vi "V1.1_UI.vi"() -> ()   [LabVIEW 2018]
uses:
  <vilib>/MakerHub/LINX/Private/Type Defs/LINX Ref.ctl
  <vilib>/MakerHub/LINX/Private/Type Defs/Platform.ctl
  <vilib>/MakerHub/LINX/Private/Type Defs/Interface.ctl
  <vilib>/MakerHub/LINX/Private/Device/Type Defs/LINX Device Config.ctl
  <vilib>/MakerHub/LINX/Private/Device/Type Defs/TCP Config.ctl
  <vilib>/MakerHub/LINX/Private/Device/Type Defs/Channels.ctl
  <vilib>/MakerHub/LINX/Public/Peripherals/Digital/Digital Write N Chans.vi
  <vilib>/MakerHub/LINX/Private/Local IO/LinxDigitalWrite.vi
  <vilib>/MakerHub/LINX/Public/Utilities/Check Channel.vi
  <vilib>/MakerHub/LINX/Public/Utilities/Open Serial.vi
  <vilib>/MakerHub/LINX/Private/Utilties/Generate Error.vi
  lib/Olympus IX BX Series/Olympus IX BX Series.lvlib
  <vilib>/MakerHub/LINX/LMH-LINX.lvlib
  lib/SOLA/LabVIEW 2015 Library (32bit)/LumencorDLL32/LumencorDLL32.lvlib
  lib/ANDOR/Andor SDK/AndorSDK.lvlib
  <vilib>/vision/NI_Vision_Development_Module.lvlib
  <userlib>/Tango_DLL/Tango_DLL.lvlib
  <userlib>/Andor SDK/Andor SDK.lvlib
  <vilib>/MakerHub/LINX/Private/Device/Device.lvlib
panel:
  in  "Export List":bool
  in  "Colormap":u16(ring) items=["Grey", "Hot"]
  in  "Format":u16(ring)=6
  in  "Path":path
  in  "Save Image":bool
  out "error out":errorcluster
  out "SOLA ID":u32
  out "TANGO ID":i32
  out "LINX Resource":T1={"IO"=enum."Remote", "Interface"=enum."TCP", "LINX Device Config"={"Interface"=enum."Serial", "COM Port"="COM13", "TCP Configuration"={"IP Address"="", "Port"=0}, "Device Family"=1, "Device ID"=1, "Device Name"="myRIO-1900", "TCP Ref"=refnum, "Channels"={"DI"=[0, 1, 2, 3, 4, 5, 6, 7, 8, 9, 10, 11, 12, 13, 14, 15, 16, 17, 18, 19, 20, 21, 22, 23, 24, 25, 26, 27, 28, 29, 30, 31, 32, 33, 34, 35, 36, 37, 38, 39, 40, 41, 42, 43, 44, 45, 46], "DO"=[0, 1, 2, 3, 4, 5, 6, 7, 8, 9, 10, 11, 12, 13, 14, 15, 16, 17, 18, 19, 20, 21, 22, 23, 24, 25, 26, 27, 28, 29, 30, 31, 32, 33, 34, 35, 36, 37, 38, 39, 40, 41, 42, 43, 44, 45, 46], "AI"=[0, 1, 2, 3, 4, 5, 6, 7, 8, 9, 10, 11], "AO"=[], "PWM"=[3, 5, 6, 9, 10], "QE"=[], "UART"=[0, 1], "I2C 2"=[0], "SPI"=[0], "CAN"=[], "Servo"=[], "AI Ref (V)"=0.0, "AI Resolution (Bits)"=0, "AO Ref (V)"=0.0, "AO Resolution (Bits)"=0}}}
  out "elements":cluster{"Button":string, "Value":dbl}[](array[cluster])
  in  "Filter":u16(ring) items=["UV ", "CFP", "GFP", "YFP", "RFP", "BF (empty)"]
  in  "Exposure":sgl=50.0 format="%#_g ms"
  out "exposure out":sgl
  out "accumulate out":sgl
  out "kinetic out":sgl
  out "Camera Temperature":sgl format="%.2f °C"
  in  "Single/\nMultiring?":bool
  in  "Image Name":string="TestIMG"
  out "Acq. Error Array":cluster{i32, string}[](array[cluster])
  in  "Live Mode":bool
  in  "Single Image":bool
  in  "Calibrate at Startup":bool
  out "keys pressed":T7(array[ring])
  in  "Position List":i32[](listbox)
  in  "Down":bool
  in  "Left":bool
  in  "Up":bool
  in  "Right":bool
  in  "Clear Last Pos":bool
  in  "Save Pos":bool
  out "Tango Success":bool
  in  "TANGO COM Port":refnum<visa-resource-name>="COM4"
  in  "SOLA COM Port":refnum<visa-resource-name>="COM5"
  in  "Valve Port (Arduino)":refnum<visa-resource-name>="COM7"
  in  "IX 81 Port":refnum<visa-resource-name>="IX2-UCB"
  out "Tango Connection\n Error":i32
  out "Y Limits":dbl[](array[numeric]) caption="Y Limits [µm]" format="%#_12f"
  out "X Limits":dbl[](array[numeric]) caption="X Limits [µm]" format="%#_10f"
  in  "TangoStep":dbl=100.0 caption="Step Width [µm]" min=0.0 format="%#_6f"
  out "Position":dbl[](array[numeric]) caption="Position [µm]" format="%#_12f"
  in  "Focus [um]":dbl format="%.3f"
  out "Upper Limit":dbl
  out "Lower Limit":dbl
  in  "Light Source":u16(ring) items=["BF - Lamp", "SOLA"]
  in  "Intensity [%]":dbl(slide) scale=0.0..100.0 scale format="%.1f"
  in  "Prism Position (1: Bi)":enum16{"Bi", "Side"}(ring)=enum."Side"
  in  "Objective":enum16{"x 4", "x 10", "x 20", "x 40", "x 100"}(ring)=enum."x 10"
  in  "Shutter":bool
  in  "Enable Lamp":bool
  in  "Lamp Type (0: Transmitted)":enum16{"Transmitted", "Reflected"}(ring)
  out "Info":string caption="String"
  out "Image":T8(plugin-control)
  in  "Flush\nReagent":u16
  in  "Flush":bool
  in  "Pump Cycles":dbl=20.0
  in  "Frequency":dbl=50.0 format="%#_3f"
  in  "Pump On":bool
  in  "Feed On":bool
  in  "Feed Cycles":i32=20
  in  "Feed\nReagent":u16=2
  in  "Ring":u16
  in  "All Rings":bool
  in  "stop":bool
  # "Initialization"
  # "Stage"
  # "X"
  # "Y"
  # "min"
  # "min"
  # "max"
  # "max"
  # "S"
  # "M"
  # "Microscope"
  # "Valve Functions"
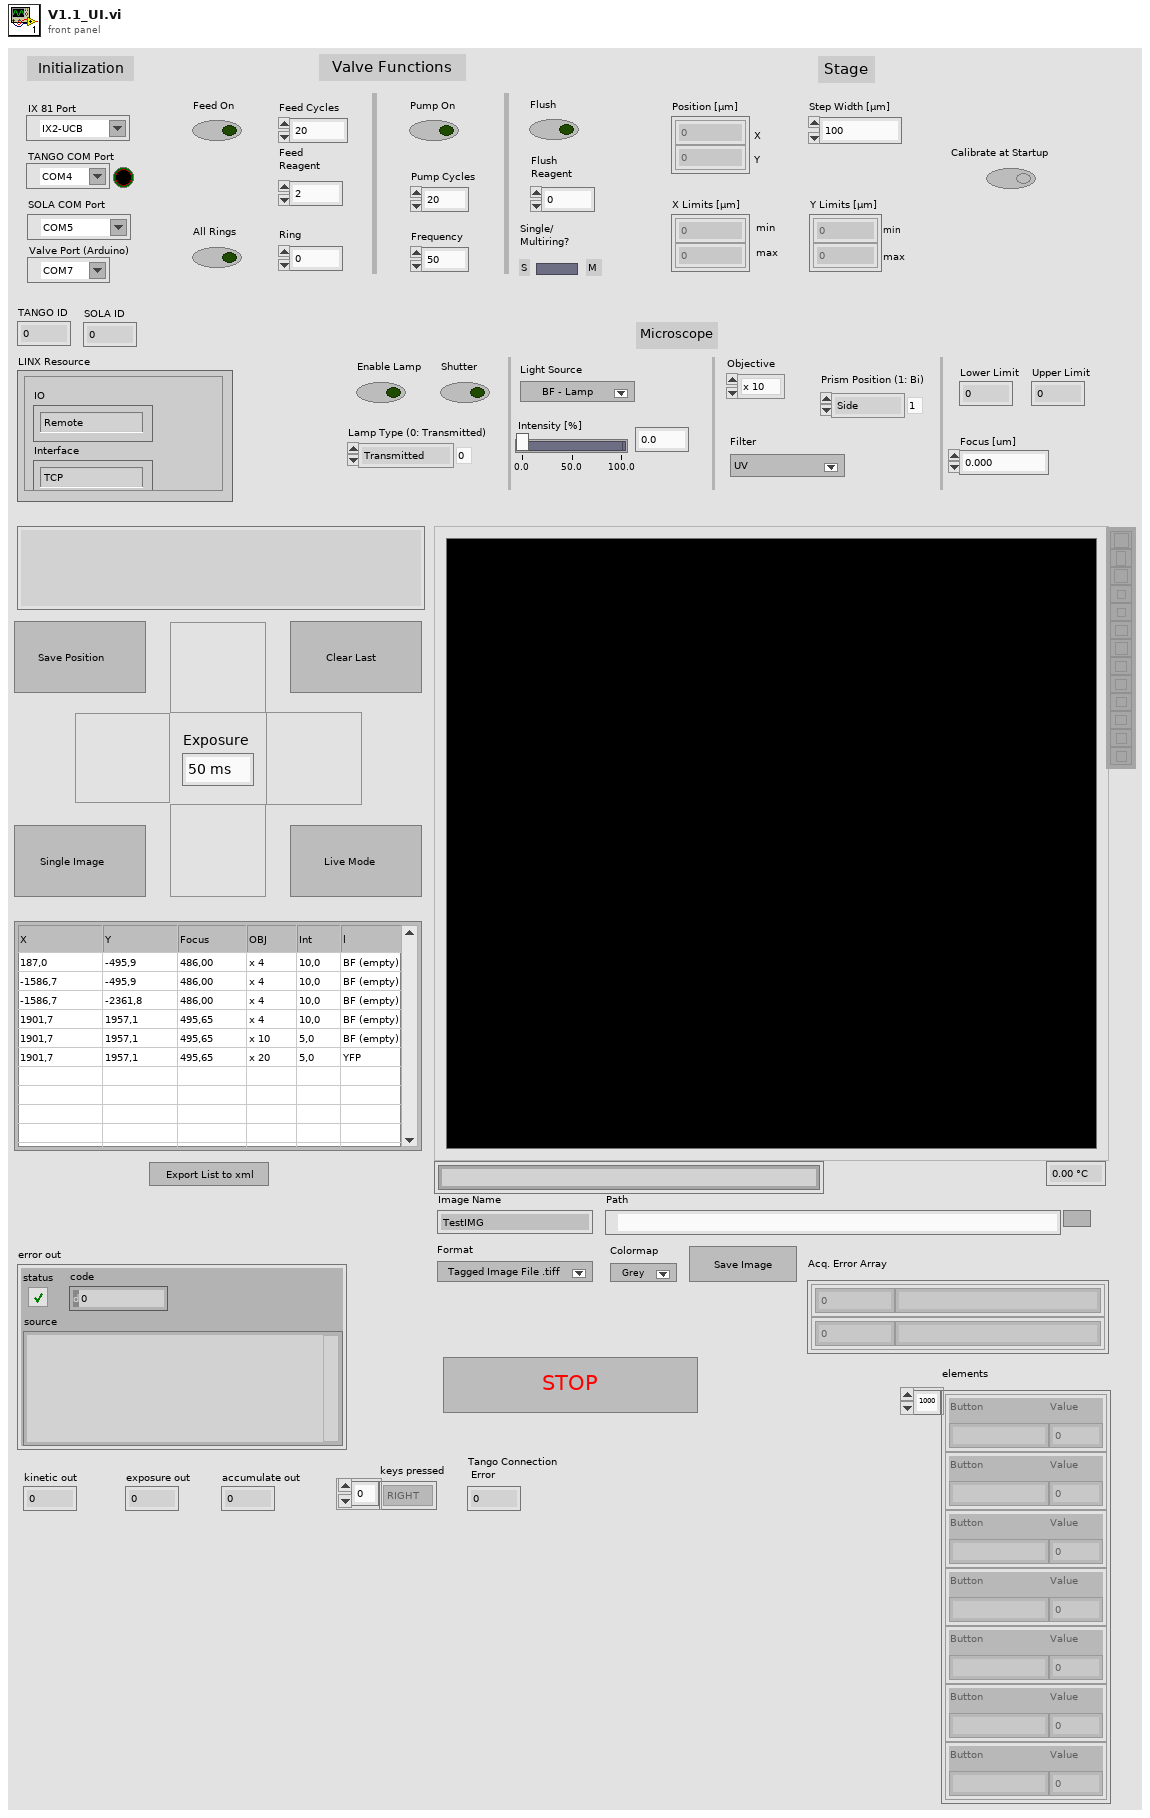
[diagram p1: front panel]
types:
  T1 = typedef "LMH-LINX.lvlib/LINX Ref.ctl" = cluster{"IO":T2, "Interface":T3, "LINX Device Config":T4}
  T2 = typedef "LMH-LINX.lvlib/Platform.ctl" = enum16{"Remote", "Local"}
  T3 = typedef "LMH-LINX.lvlib/Interface.ctl" = enum16{"Serial", "TCP"}
  T4 = typedef "LMH-LINX.lvlib/Device.lvlib/LINX Device Config.ctl" = cluster{"Interface":T3, "COM Port":refnum<visa-resource-name>, "TCP Configuration":T5, "Device Family":u8, "Device ID":u8, "Device Name":string, "TCP Ref":refnum<k5>, "Channels":T6}
  T5 = typedef "LMH-LINX.lvlib/Device.lvlib/TCP Config.ctl" = cluster{"IP Address":string, "Port":u16}
  T6 = typedef "LMH-LINX.lvlib/Channels.ctl" = cluster{"DI":u8[], "DO":u8[], "AI":u8[], "AO":u8[], "PWM":u8[], "QE":u8[], "UART":u8[], "I2C 2":u8[], "SPI":u8[], "CAN":u8[], "Servo":u8[], "AI Ref (V)":dbl, "AI Resolution (Bits)":u8, "AO Ref (V)":dbl, "AO Resolution (Bits)":u8}
  T7 = enum16{"0", "1", "2", "3", "4", "5", "6", "7", "8", "9", "A", "B", "C", "D", "E", "F", "G", "H", "I", "J", "K", "L", "M", "N", "O", "P", "Q", "R", "S", "T", "U", "V", "W", "X", "Y", "Z", "F1", "F2", "F3", "F4", "F5", "F6", "F7", "F8", "F9", "F10", "F11", "F12", "F13", "F14", "F15", "ADD", "BACK", "BACKSLASH", "CAPITAL", "COMMA", "DECIMAL", "DELETE", "DIVIDE", "DOWN", "END", "EQUALS", "ESCAPE", "GRAVE (`)", "HOME", "INSERT", "LBRACKET", "LCONTROL", "LEFT", "L ALT", "LSHIFT", "LWIN", "MINUS", "MULTIPLY", "NEXT", "NUMLOCK", "NUMPAD_0", "NUMPAD_1", "NUMPAD_2", "NUMPAD_3", "NUMPAD_4", "NUMPAD_5", "NUMPAD_6", "NUMPAD_7", "NUMPAD_8", "NUMPAD_9", "PAUSE", "PERIOD", "PRIOR (PG UP)", "RBRACKET", "RCONTROL", "RETURN", "RIGHT", "R ALT", "RSHIFT", "RWIN", "SCROLL", "SEMICOLON", "SLASH", "SPACE", "SUBTRACT", "TAB", "UP", "ENTER (num pad)", "' (quote)"}[]
  T8 = typedef "IMAQ Image.ctl" = refnum<image>
  T9 = enum8{"Enabled", "Disabled", "Disabled and Grayed Out"}
  T10 = enum32{"UV", "CFP", "GFP", "YFP", "RFP", "BF (empty)"}
  T11 = typedef "Image Type" = u32
  T12 = cluster{"pdX out":dbl, "pdY out":dbl, dbl, string, string, "Intensity [%]":dbl}
  T13 = cluster{"pdX out":dbl, "pdY out":dbl, dbl, string, string, "Intensity [%]":dbl}[]
  T14 = cluster{string, "NewVal":enum16{"x 4", "x 10", "x 20", "x 40", "x 100"}}
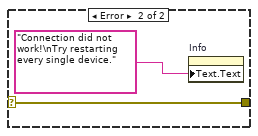
[diagram p2: hidden frame]
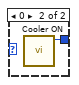
[diagram p3: hidden frame]
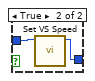
[diagram p4: hidden frame]
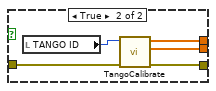
[diagram p5: hidden frame]
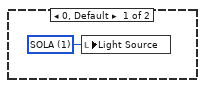
[diagram p6: hidden frame]
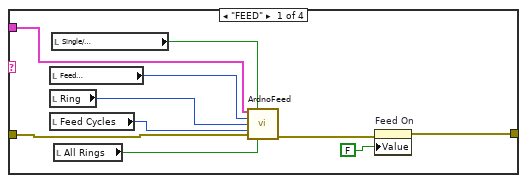
[diagram p7: hidden frame]
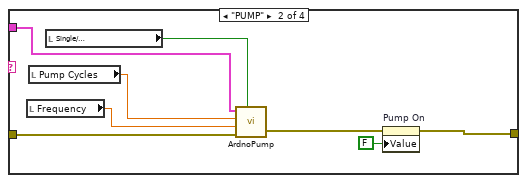
[diagram p8: hidden frame]
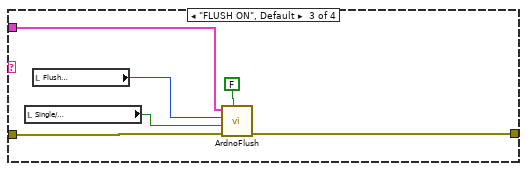
[diagram p9: hidden frame]
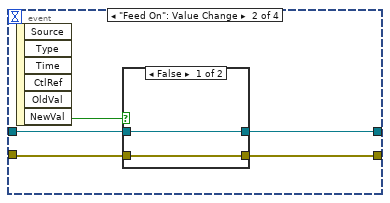
[diagram p10: hidden frame]
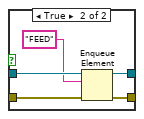
[diagram p11: hidden frame]
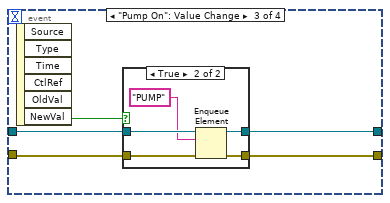
[diagram p12: hidden frame]
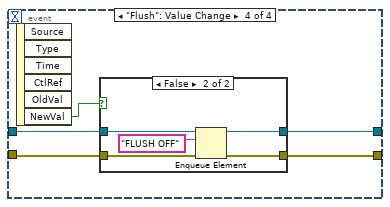
[diagram p14: hidden frame]
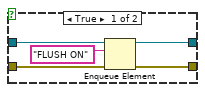
[diagram p15: hidden frame]
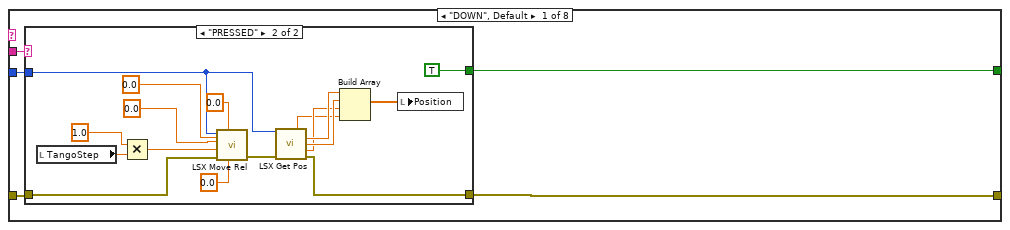
[diagram p16: hidden frame]
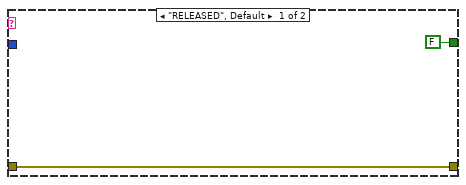
[diagram p17: hidden frame]
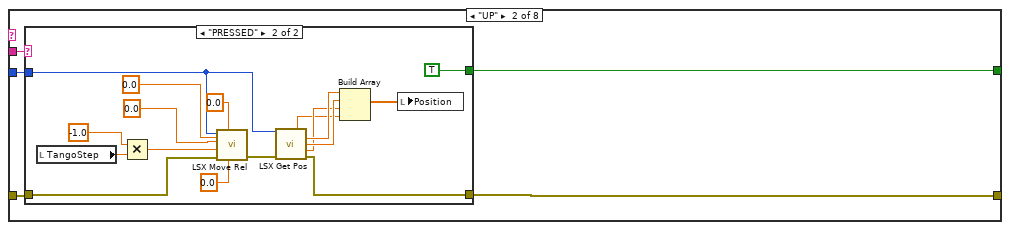
[diagram p18: hidden frame]
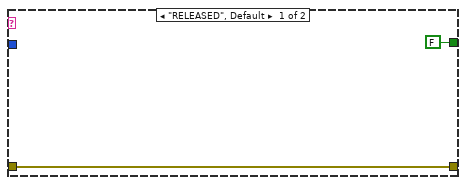
[diagram p19: hidden frame]
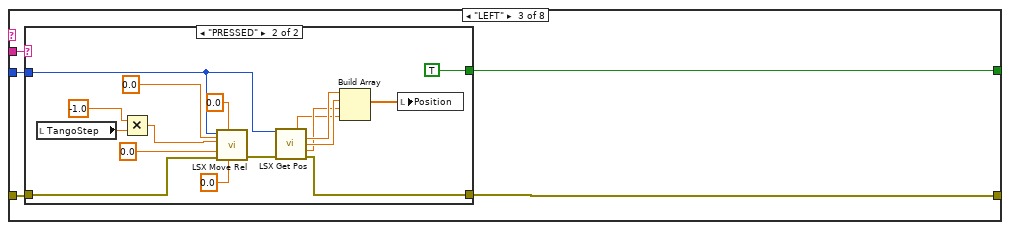
[diagram p20: hidden frame]
diagram:
  n1 = flat-sequence {
    tunnel: [w15] -> w2
    tunnel: w2 -> [w119]
    tunnel: [w115] -> w1
    tunnel: w1 -> [w228]
    tunnel: [w233] -> w5
    tunnel: w5 -> [w1109]
    tunnel: [w1108] -> w4
    tunnel: w4 -> [w1135]
    tunnel: [w1135] -> w3
    frame #0 {
      # "Connection String"
      n2 = local write "Info"("Connecting..." ("Info")) -> ()
    }
    frame #1 {
      w29 = 2  # Device Number (1: Condensor, Objective Lamp,Shutter 2: Z-Motion, Autofocus)
      w32 = 1  # Device Number (1: Condensor, Objective Lamp,Shutter 2: Z-Motion, Autofocus)
      # "Establishing Connections To All Devices"
      n3 = local read "Valve Port (Arduino)"() -> (w27:refnum<visa-resource-name>)
      n4 = property on="SOLA COM Port" class="VISAName"() -> ("Text.Text"=w24:string)  [unwired: 2 in, 2 out]
      n5 = local read "TANGO COM Port"() -> (w11:refnum<visa-resource-name>)
      n6 = local read "IX 81 Port"() -> (w28:refnum<visa-resource-name>)
      n7 = Scan From String(format string="COM%d", input string=w24) -> (output 1=w22:i32)  [unwired: 3 in, 3 out]
      n8 = Decrement(x=w22) -> (x-1=w21:i32)
      n9 = call-poly <vilib>:"Open.vi"("Serial Port"=w27) -> ("Error Out"=w25:errorcluster, "LINX Resource"=→"LINX Resource":T1)  [unwired: 8 in, 1 out]
      n10 = call "Initialize.vi"("VISA Resource Name"=w28) -> ("VISA Resource Name Out"=w33:refnum<visa-resource-name>, "error out"=w34:errorcluster)  [unwired: 13 in]
      n11 = call "lm Init.vi"("LETypeStr"="SOLA", "ComPort"=w21) -> ("error out"=w19:errorcluster, "function return"=→"SOLA ID":u32)  [unwired: 7 in, 1 out]
      n12 = call "AndorCreaterErrorCluster.vi"() -> ("Array"=w7:cluster{i32, string}[])  [unwired: 11 in]
      n13 = call "TangoConnect.vi"("Tango Com"=w11) -> ("error out"=w10:errorcluster, "success"=w8:bool, "plLSID out"=→"TANGO ID":i32)  [unwired: 7 in, 1 out]
      n14 = call "Initialize.vi"("dir"="C:\\Users\\e14user\\Documents\\LabVIEW software\\GitRepo\\lib\\ANDOR\\Libraries") -> ("function return"=w17:u32)  [unwired: 9 in, 1 out]
      n15 = call "Login Device.vi"("error in (no error)"=w34, "Device Number (1)"=w32, "VISA Resource Name"=w33) -> ("error out"=w30:errorcluster, "VISA Resource Name Out"=w31:refnum<visa-resource-name>)  [unwired: 7 in]
      n16 = call "Login Device.vi"("error in (no error)"=w30, "Device Number (1)"=w29, "VISA Resource Name"=w31) -> ("error out"=w26:errorcluster)  [unwired: 7 in, 1 out]
      n17 = local write "Tango Success"(w8) -> ()
      n18 = property on="Tango Success" class="Bool (strict)"("Colors [4]"=cluster{u32, u32}[] [{16711680, 0}, {65280, 0}, {6710886, 0}, {6710886, 0}]) -> ()  [unwired: 2 in, 2 out]
      n19 = call "AndorReturn2Error.vi"("Error List"=w7, "Camera return"=w17) -> ("error out"=w16:errorcluster)  [unwired: 8 in, 1 out]
      n20 = Merge Errors(w26, w25, w19, w10, w16) -> (w14:errorcluster)
      n21 = case shown="No Error" w14 {
        selector: w14 -> [w36 w39]
        tunnel: [w36 w39] -> w15
        frame No Error {
          n22 = property on="Info" class="Str"("Text.Text"="Connection finished!") -> ()  [unwired: 2 in, 2 out]
        }
        frame Error {
          n23 = property on="Info" class="Str"("Text.Text"="Connection did not work!\nTry restarting every single device.") -> ()  [unwired: 2 in, 2 out]
        }
      }
    }
    frame #2 {
      w104 = 0  # openingtime
      w102 = 0  # Auto Mode
      w101 = 1  # TTL High to open
      w103 = 0  # closingtime
      w100 = 0  # Internal Trigger
      w98 = 1  # Single Scan
      w99 = 4  # Image Read
      # "Initializing Devices With (Config File)"
      n24 = local read "Calibrate at Startup"() -> (w124:bool)
      n25 = local read "IX 81 Port"() -> (w194:refnum<visa-resource-name>)
      n26 = call "AndorCreaterErrorCluster.vi"() -> ("Array"=w72:cluster{i32, string}[])  [unwired: 11 in]
      n27 = call "Is Cooler On.vi"() -> ("function return"=w87:u32, "iCoolerStatus out"=w88:i32)  [unwired: 10 in]
      n28 = call "lm Color Level.vi"("error in (no error)"=w119, "str_Level"="0", "str_Color"="WHITE") -> ("error out"=w198:errorcluster, "str_Color out"=w199:string)  [unwired: 6 in, 1 out]
      n29 = call "Set Active Objective.vi"("error in (no error)"=w119, "Objective Number (1)"=1, "Device Number (1)"=1, "VISA Resource Name"=w194) -> ("error out"=w141:errorcluster, "VISA Resource Name Out"=w142:refnum<visa-resource-name>)  [unwired: 6 in]
      n30 = call "AndorReturn2Error.vi"("Error List"=w72, "Camera return"=w87) -> ("error out"=w70:errorcluster, "Error List out"=w71:cluster{i32, string}[])  [unwired: 8 in]
      n31 = call "lm Color Enable.vi"("error in (no error)"=w198, "str_State"="OFF", "str_Color"=w199) -> ("error out"=w112:errorcluster)  [unwired: 6 in, 2 out]
      n32 = case shown="False" w124 {
        tunnel: [w207 w214] -> w111
        tunnel: w119 -> [w207 w210]
        tunnel: [dbl[] [0.0, 80674.8] ("Y Limits") w213] -> w122
        tunnel: [dbl[] [0.0, 120822.0] ("X Limits") w212] -> w123
        frame False {
        }
        frame True {
          n33 = local read "TANGO ID"() -> (w211:i32)
          n34 = call "TangoCalibrate.vi"("error in (no error)"=w210, "plLSID in"=w211) -> ("error out"=w214:errorcluster, "X Limits"=w212:dbl[], "Y Limits"=w213:dbl[])  [unwired: 7 in]
        }
      }
      n35 = case shown="1, Default" w88 {
        tunnel: [u32 20002 ("function return") w203] -> w86
        frame 1, Default {
        }
        frame 0 {
          n36 = call "Cooler ON.vi"() -> ("function return"=w203:u32)  [unwired: 11 in]
        }
      }
      n37 = call "OlympusQuery.vi"("error in (no error)"=w141, "String"="SW OFF", "VISA Resource Name In"=w142) -> ("error out"=w145:errorcluster, "VISA Resource Name Out"=w146:refnum<visa-resource-name>)  [unwired: 6 in, 1 out]
      n38 = call "OlympusQuery.vi"("error in (no error)"=w145, "String"="LMPSW?", "VISA Resource Name In"=w146) -> ("error out"=w140:errorcluster, "Result"=w173:string, "VISA Resource Name Out"=w191:refnum<visa-resource-name>)  [unwired: 6 in]
      n39 = call "AndorReturn2Error.vi"("error in (no error)"=w70, "Error List"=w71, "Camera return"=w86) -> ("error out"=w69:errorcluster, "Error List out"=w43:cluster{i32, string}[])  [unwired: 7 in]
      n40 = Equal?(x=w173, y="ON") -> (x = y?=w139:bool)
      n41 = local write "Enable Lamp"(w139) -> ()
      n42 = call "OlympusQuery.vi"("error in (no error)"=w140, "String"="LMP?", "VISA Resource Name In"=w191) -> ("error out"=w137:errorcluster, "Result"=w148:string, "VISA Resource Name Out"=w190:refnum<visa-resource-name>)  [unwired: 6 in]
      n43 = call "Set Temperature.vi"("temperature"=-60) -> ()  [unwired: 10 in, 1 out]
      n44 = Decimal String To Number(string=w148, default (0L)=0.0 ("default (0 I32)")) -> (number=w150:dbl)  [unwired: 1 in, 1 out]
      n45 = local read "LINX Resource"() -> (w121:T1)
      n46 = local write "Y Limits"(w122) -> ()
      n47 = local write "X Limits"(w123) -> ()
      n48 = Divide(x=w150, y=1.2 ("x")) -> (x/y=w138:dbl)
      n49 = local write "Intensity [%]"(w138) -> ()
      n50 = call "ArdnoValve2Linx.vi"("error in (no error)"=w119, "Valve (A1-C8),\n comma separated"="A1,A2,A3,A4,A5,A6,A7,A8,B1,B2,B3,B4,B5,B6,B7,B8,C1,C2,C3,C4,C5,C6,C7,C8" ("Valve (A1-C8),\n comma separated")) -> ("error out"=w118:errorcluster, "Array"=w117:bool[], "Array 2"=w116:i32[])  [unwired: 7 in]
      n51 = call "Get Fastest Recommended VS Speed.vi"() -> ("function return"=w73:u32, "speed out"=w106:sgl, "index out"=w109:i32)  [unwired: 9 in]
      n52 = call "OlympusQuery.vi"("error in (no error)"=w137, "String"="SHUT1?", "VISA Resource Name In"=w190) -> ("error out"=w135:errorcluster, "Result"=w171:string, "VISA Resource Name Out"=w188:refnum<visa-resource-name>)  [unwired: 6 in]
      n53 = call-poly <vilib>:"Digital Write.vi"("Error In"=w118, "Values"=w117, "DO Channels"=w116, "LINX Resource"=w121) -> ("Error Out"=w113:errorcluster)  [unwired: 6 in, 1 out]
      n54 = Equal?(x=w171, y="OUT") -> (x = y?=w136:bool)
      n55 = local write "Shutter"(w136) -> ()
      n56 = call "AndorReturn2Error.vi"("error in (no error)"=w69, "Error List"=w43, "Camera return"=w73) -> ("error out"=w68:errorcluster, "Error List out"=w44:cluster{i32, string}[])  [unwired: 7 in]
      n57 = call "Get VS Speed.vi"() -> ("speed out"=w107:sgl, "function return"=w74:u32)  [unwired: 10 in]
      n58 = call "OlympusQuery.vi"("error in (no error)"=w135, "String"="LMPSEL?", "VISA Resource Name In"=w188) -> ("error out"=w132:errorcluster, "Result"=w169:string, "VISA Resource Name Out"=w133:refnum<visa-resource-name>)  [unwired: 6 in]
      n59 = Greater Or Equal?(x=w106, y=w107) -> (x >= y?=w108:bool)
      n60 = call "AndorReturn2Error.vi"("error in (no error)"=w68, "Error List"=w44, "Camera return"=w74) -> ("error out"=w67:errorcluster, "Error List out"=w45:cluster{i32, string}[])  [unwired: 7 in]
      n61 = Equal?(x=w169, y="DIA") -> (x = y?=w167:bool)
      n62 = Not(x=w167) -> (.not. x?=w166:bool)
      n63 = case shown="False" w108 {
        tunnel: w109 -> [_ w206]
        tunnel: [u32 20002 ("function return") w205] -> w75
        frame False {
        }
        frame True {
          n64 = call "Set VS Speed.vi"("index"=w206) -> ("function return"=w205:u32)  [unwired: 10 in]
        }
      }
      n65 = Boolean To (0,1)(Boolean=w166) -> (0, 1=w134:i16)
      n66 = local write "Lamp Type (0: Transmitted)"(w134) -> ()
      n67 = call "OlympusQuery.vi"("error in (no error)"=w132, "String"="MU?", "VISA Resource Name In"=w133) -> ("error out"=w131:errorcluster, "Result"=w165:string, "VISA Resource Name Out"=w144:refnum<visa-resource-name>)  [unwired: 6 in]
      n68 = call "AndorReturn2Error.vi"("error in (no error)"=w67, "Error List"=w45, "Camera return"=w75) -> ("error out"=w66:errorcluster, "Error List out"=w46:cluster{i32, string}[])  [unwired: 7 in]
      n69 = Decimal String To Number(string=w165) -> (number=w164:i32)  [unwired: 2 in, 1 out]
      n70 = call "Get Temperature F.vi"() -> ("function return"=w76:u32, "temperature out"=w105:sgl)  [unwired: 10 in]
      n71 = Decrement(x=w164) -> (x-1=w143:i32)
      n72 = case shown="5" w143 {
        frame 0, Default {
          w215 = u16 1 items=["BF - Lamp", "SOLA"] ("Light Source")
          n73 = local write "Light Source"(w215) -> ()
        }
        frame 5 {
          w216 = u16 0 items=["BF - Lamp", "SOLA"] ("Light Source")
          n74 = local write "Light Source"(w216) -> ()
        }
      }
      n75 = local write "Filter"(w143) -> ()
      n76 = call "AndorReturn2Error.vi"("error in (no error)"=w66, "Error List"=w46, "Camera return"=w76) -> ("error out"=w65:errorcluster, "Error List out"=w47:cluster{i32, string}[])  [unwired: 7 in]
      n77 = local write "Camera Temperature"(w105) -> ()
      n78 = call "OlympusQuery.vi"("error in (no error)"=w131, "String"="OB?", "VISA Resource Name In"=w144) -> ("error out"=w129:errorcluster, "Result"=w163:string, "VISA Resource Name Out"=w183:refnum<visa-resource-name>)  [unwired: 6 in]
      n79 = Decimal String To Number(string=w163) -> (number=w162:i32)  [unwired: 2 in, 1 out]
      n80 = Decrement(x=w162) -> (x-1=w130:i32)
      n81 = call "Set Read Mode.vi"("mode"=w99) -> ("function return"=w77:u32)  [unwired: 10 in]
      n82 = local write "Objective"(w130) -> ()
      n83 = call "AndorReturn2Error.vi"("error in (no error)"=w65, "Error List"=w47, "Camera return"=w77) -> ("error out"=w64:errorcluster, "Error List out"=w48:cluster{i32, string}[])  [unwired: 7 in]
      n84 = local write "Lower Limit"(10.0 ("Upper Limit")) -> ()
      n85 = call "OlympusQuery.vi"("error in (no error)"=w129, "String"="PRISM?", "VISA Resource Name In"=w183) -> ("error out"=w128:errorcluster, "Result"=w161:string, "VISA Resource Name Out"=w182:refnum<visa-resource-name>)  [unwired: 6 in]
      n86 = Decimal String To Number(string=w161) -> (number=w160:i32)  [unwired: 2 in, 1 out]
      n87 = call "Set Shutter.vi"("openingtime"=w104, "closingtime"=w103, "mode"=w102, "typ"=w101) -> ("function return"=w78:u32)  [unwired: 7 in]
      n88 = Decrement(x=w160) -> (x-1=w127:i32)
      n89 = local write "Prism Position (1: Bi)"(w127) -> ()
      n90 = call "OlympusQuery.vi"("error in (no error)"=w128, "Device Number\n(1: -Condensor\n     - Objective\n     - Lamp\n     - Shutter\n2: - Z-Motion\n   - Autofocus)"=2 ("Device Number\n(1: -Condensor\n     - Objective\n     - Lamp\n     - Shutter\n2: - Z-Motion\n   - Autofocus)"), "String"="FARLMT 10", "VISA Resource Name In"=w182) -> ("error out"=w179:errorcluster, "VISA Resource Name Out"=w180:refnum<visa-resource-name>)  [unwired: 5 in, 1 out]
      n91 = call "AndorReturn2Error.vi"("error in (no error)"=w64, "Error List"=w48, "Camera return"=w78) -> ("error out"=w63:errorcluster, "Error List out"=w49:cluster{i32, string}[])  [unwired: 7 in]
      n92 = local write "Upper Limit"(3000000.0 ("default (0 I32)")) -> ()
      n93 = call "Set Trigger Mode.vi"("mode"=w100) -> ("function return"=w79:u32)  [unwired: 10 in]
      n94 = call "AndorReturn2Error.vi"("error in (no error)"=w63, "Error List"=w49, "Camera return"=w79) -> ("error out"=w62:errorcluster, "Error List out"=w50:cluster{i32, string}[])  [unwired: 7 in]
      n95 = call "OlympusQuery.vi"("error in (no error)"=w179, "Device Number\n(1: -Condensor\n     - Objective\n     - Lamp\n     - Shutter\n2: - Z-Motion\n   - Autofocus)"=2 ("Device Number\n(1: -Condensor\n     - Objective\n     - Lamp\n     - Shutter\n2: - Z-Motion\n   - Autofocus)"), "String"="NEARLMT 3000000", "VISA Resource Name In"=w180) -> ("error out"=w176:errorcluster, "VISA Resource Name Out"=w177:refnum<visa-resource-name>)  [unwired: 5 in, 1 out]
      n96 = call "Set Acquisition Mode.vi"("mode"=w98) -> ("function return"=w80:u32)  [unwired: 10 in]
      n97 = call "OlympusQuery.vi"("error in (no error)"=w176, "Device Number\n(1: -Condensor\n     - Objective\n     - Lamp\n     - Shutter\n2: - Z-Motion\n   - Autofocus)"=2 ("Device Number\n(1: -Condensor\n     - Objective\n     - Lamp\n     - Shutter\n2: - Z-Motion\n   - Autofocus)"), "String"="POS?", "VISA Resource Name In"=w177) -> ("error out"=w154:errorcluster, "Result"=w155:string, "VISA Resource Name Out"=w153:refnum<visa-resource-name>)  [unwired: 5 in]
      n98 = call "AndorReturn2Error.vi"("error in (no error)"=w62, "Error List"=w50, "Camera return"=w80) -> ("error out"=w61:errorcluster, "Error List out"=w51:cluster{i32, string}[])  [unwired: 7 in]
      n99 = call "Set Frame Transfer Mode.vi"("mode"=1) -> ("function return"=w81:u32)  [unwired: 10 in]
      n100 = Decimal String To Number(string=w155, default (0L)=0.0 ("default (0 I32)")) -> (number=w41:dbl)  [unwired: 1 in, 1 out]
      n101 = call "AndorReturn2Error.vi"("error in (no error)"=w61, "Error List"=w51, "Camera return"=w81) -> ("error out"=w60:errorcluster, "Error List out"=w52:cluster{i32, string}[])  [unwired: 7 in]
      n102 = Divide(x=w41, y=1000.0) -> (x/y=w40:dbl)
      n103 = call "Set Number Accumulations.vi"("number"=1) -> ("function return"=w82:u32)  [unwired: 10 in]
      n104 = call "Configure Jog.vi"("VISA Resource Name"=w153, "Device Number (1)"=2, "Enabled (False)"=TRUE, "error in (no error)"=w154) -> ("error out"=w114:errorcluster)  [unwired: 10 in, 1 out]
      n105 = local write "Focus [um]"(w40) -> ()
      n106 = local read "Exposure"() -> (w94:sgl)
      n107 = call "AndorReturn2Error.vi"("error in (no error)"=w60, "Error List"=w52, "Camera return"=w82) -> ("error out"=w59:errorcluster, "Error List out"=w53:cluster{i32, string}[])  [unwired: 7 in]
      n108 = call "Set Number Kinetics.vi"("number"=1) -> ("function return"=w83:u32)  [unwired: 10 in]
      n109 = call "AndorReturn2Error.vi"("error in (no error)"=w59, "Error List"=w53, "Camera return"=w83) -> ("error out"=w58:errorcluster, "Error List out"=w54:cluster{i32, string}[])  [unwired: 7 in]
      n110 = Divide(x=w94, y=sgl 1000.0) -> (x/y=w93:sgl)
      n111 = call "Set Exposure Time.vi"("time"=w93) -> ("function return"=w84:u32)  [unwired: 10 in]
      n112 = call "AndorReturn2Error.vi"("error in (no error)"=w58, "Error List"=w54, "Camera return"=w84) -> ("error out"=w57:errorcluster, "Error List out"=w55:cluster{i32, string}[])  [unwired: 7 in]
      n113 = call "Get Acquisition Timings.vi"() -> ("kinetic out"=w91:sgl, "accumulate out"=w89:sgl, "exposure out"=w90:sgl, "function return"=w85:u32)  [unwired: 8 in]
      n114 = call "AndorReturn2Error.vi"("error in (no error)"=w57, "Error List"=w55, "Camera return"=w85) -> ("error out"=w56:errorcluster)  [unwired: 7 in, 1 out]
      n115 = local write "exposure out"(w90) -> ()
      n116 = local write "accumulate out"(w89) -> ()
      n117 = local write "kinetic out"(w91) -> ()
      n118 = Merge Errors(w114, w113, w112, w111, w56) -> (w115:errorcluster)
    }
    frame #3 {
      w229 = ""  # Button
      w239 = ""  # Button
      n119 = flat-sequence {
        frame #0 {
          # "Event Handling for Single, Live Mode and Exposure Time Changes"
          n120 = call "AndorCreaterErrorCluster.vi"() -> ("Array"=w632:cluster{i32, string}[])  [unwired: 11 in]
          n121 = while {
            tunnel: 0 -> [w641]
            tunnel: w632 -> [w636]
            shift-right: [w638] -> _
            shift-left: FALSE -> [w639]
            stop <- w635 stop-if-true
            n122 = event shown="[1] \"Save Image\": Value Change" {
              selector: _ -> [_ _ _ _ _]
              dyn-events: _ -> [_ _ _ _ _]
              timeout: w641 -> [_ _ _ _ _]
              tunnel: w636 -> [_ w646 _ w785 _]
              tunnel: [w643 FALSE ("NewVal") w768 FALSE w855] -> w640
              tunnel: w639 -> [w643 _ w768 _ _]
              event Timeout {
                n123 = event-data() -> ()  [unwired: 1 in, 3 out]
              }
              event "Save Image": Value Change {
                n124 = event-data() -> ("NewVal"=w649:bool)  [unwired: 1 in, 5 out]
                n125 = local read "Image Name"() -> (w653:string)
                n126 = property on="Path" class="Path"() -> ("Value"=w651:path)  [unwired: 2 in, 2 out]
                n127 = Not(x=w649) -> (.not. x?=w648:bool)
                n128 = Empty String/Path?(string/path=w651) -> (empty?=w652:bool)
                n129 = Empty String/Path?(string/path=w653) -> (empty?=w654:bool)
                n130 = Build Array(w648, w652, w654) -> (w650:bool[])
                n131 = Or Array Elements(Boolean array=w650) -> (logical OR=w647:bool)
                n132 = case shown="False" w647 {
                  tunnel: w646 -> [w659 _]
                  frame False {
                    n133 = flat-sequence {
                      tunnel: w659 -> [w665]
                      tunnel: [w664] -> w657
                      tunnel: w657 -> [w667]
                      tunnel: [w667] -> w656
                      tunnel: w659 -> [w677]
                      tunnel: [w676] -> w658
                      tunnel: w656 -> [w675]
                      tunnel: [w675] -> w655
                      tunnel: w658 -> [w765]
                      tunnel: w655 -> [w764]
                      frame #0 {
                        w662 = 1  # Single Scan
                        w663 = 4  # Image Read
                        n134 = call "Set Number Accumulations.vi"("number"=1) -> ()  [unwired: 10 in, 1 out]
                        n135 = call "Set Number Kinetics.vi"("number"=1) -> ()  [unwired: 10 in, 1 out]
                        n136 = call "Set Acquisition Mode.vi"("mode"=w662) -> ()  [unwired: 10 in, 1 out]
                        n137 = call "Set Read Mode.vi"("mode"=w663) -> ()  [unwired: 10 in, 1 out]
                      }
                      frame #1 {
                        n138 = call "Start Acquisition.vi"() -> ("function return"=w666:u32)  [unwired: 11 in]
                        n139 = call "ConvertErrCodeToMessage.vi"("function return"=w666, "Array"=w665) -> ("Element Return"=w664:cluster{i32, string})  [unwired: 8 in, 1 out]
                      }
                      frame #2 {
                        n140 = while {
                          stop <- w668 stop-if-true
                          n141 = call "Get Status.vi"() -> ("function return"=w671:u32, "status out"=w672:i32)  [unwired: 10 in]
                          n142 = Equal?(x=w671, y=20002 ("x")) -> (x = y?=w674:bool)
                          n143 = Equal?(x=20073 ("status out"), y=w672) -> (x = y?=w673:bool)
                          n144 = And(x=w673, y=w674) -> (x .and. y?=w668:bool)
                        }
                      }
                      frame #3 {
                        n145 = local read "Format"() -> (w680:u16)
                        n146 = local read "Image Name"() -> (w678:string)
                        n147 = local read "Path"() -> (w679:path)
                        n148 = case shown="6, Default" w680 {
                          tunnel: w679 -> [w691 w702 w712 w722 w732 w741 w754 _]
                          tunnel: w678 -> [w690 w701 w711 w721 w731 w740 w753 _]
                          tunnel: w677 -> [w686 w695 w707 w717 w727 w736 w749 _]
                          tunnel: [w685 w694 w706 w716 w726 w735 w748 w760] -> w676
                          frame 0 {
                            n149 = local read "Colormap"() -> (w682:u16)
                            n150 = Concatenate Strings(w690, ".bmp" ("string")) -> (w688:string)
                            n151 = case shown="0, Default" w682 {
                              tunnel: ["C:\\Users\\e14user\\Documents\\LabVIEW software\\GitRepo\\config\\Palettes\\Grey.pal" "C:\\Users\\e14user\\Documents\\LabVIEW software\\GitRepo\\config\\Palettes\\Hot.pal"] -> w681
                              frame 0, Default {
                              }
                              frame 1 {
                              }
                            }
                            n152 = Build Path(base path=w691, name or relative path=w688) -> (appended path=w687:path)
                            n153 = Path To String(path=w687) -> (string=w683:string)
                            n154 = call <userlib>:"Save As Bmp.vi"("palette"=w681, "path"=w683) -> ("function return"=w684:u32)  [unwired: 6 in, 3 out]
                            n155 = call "ConvertErrCodeToMessage.vi"("function return"=w684, "Array"=w686) -> ("Element Return"=w685:cluster{i32, string})  [unwired: 8 in, 1 out]
                          }
                          frame 1 {
                            n156 = Concatenate Strings(w701, ".sif" ("string")) -> (w699:string)
                            n157 = Build Path(base path=w702, name or relative path=w699) -> (appended path=w697:path)
                            n158 = Path To String(path=w697) -> (string=w698:string)
                            n159 = call <userlib>:"Save As Sif.vi"("path"=w698) -> ("function return"=w696:u32)  [unwired: 8 in, 2 out]
                            n160 = call "ConvertErrCodeToMessage.vi"("function return"=w696, "Array"=w695) -> ("Element Return"=w694:cluster{i32, string})  [unwired: 8 in, 1 out]
                          }
                          frame 2 {
                            n161 = Concatenate Strings(w711, ".edf" ("string")) -> (w709:string)
                            n162 = Build Path(base path=w712, name or relative path=w709) -> (appended path=w708:path)
                            n163 = Path To String(path=w708) -> (string=w704:string)
                            n164 = call <userlib>:"Save As EDF.vi"("iMode"=0, "szPath"=w704) -> ("function return"=w705:u32)  [unwired: 7 in, 2 out]
                            n165 = call "ConvertErrCodeToMessage.vi"("function return"=w705, "Array"=w707) -> ("Element Return"=w706:cluster{i32, string})  [unwired: 8 in, 1 out]
                          }
                          frame 3 {
                            n166 = Concatenate Strings(w721, ".fits" ("string")) -> (w719:string)
                            n167 = Build Path(base path=w722, name or relative path=w719) -> (appended path=w718:path)
                            n168 = Path To String(path=w718) -> (string=w715:string)
                            n169 = call <userlib>:"Save As FITS.vi"("typ"=1, "szFileTitle"=w715) -> ("function return"=w714:u32)  [unwired: 7 in, 2 out]
                            n170 = call "ConvertErrCodeToMessage.vi"("function return"=w714, "Array"=w717) -> ("Element Return"=w716:cluster{i32, string})  [unwired: 8 in, 1 out]
                          }
                          frame 4 {
                            n171 = Concatenate Strings(w731, ".raw" ("string")) -> (w729:string)
                            n172 = Build Path(base path=w732, name or relative path=w729) -> (appended path=w728:path)
                            n173 = Path To String(path=w728) -> (string=w724:string)
                            n174 = call <userlib>:"Save As Raw.vi"("typ"=3, "szFileTitle"=w724) -> ("function return"=w725:u32)  [unwired: 7 in, 2 out]
                            n175 = call "ConvertErrCodeToMessage.vi"("function return"=w725, "Array"=w727) -> ("Element Return"=w726:cluster{i32, string})  [unwired: 8 in, 1 out]
                          }
                          frame 5 {
                            n176 = Concatenate Strings(w740, ".spc" ("string")) -> (w738:string)
                            n177 = Build Path(base path=w741, name or relative path=w738) -> (appended path=w737:path)
                            n178 = Path To String(path=w737) -> (string=w733:string)
                            n179 = call <userlib>:"Save As SPC.vi"("path"=w733) -> ("function return"=w734:u32)  [unwired: 8 in, 2 out]
                            n180 = call "ConvertErrCodeToMessage.vi"("function return"=w734, "Array"=w736) -> ("Element Return"=w735:cluster{i32, string})  [unwired: 8 in, 1 out]
                          }
                          frame 6, Default {
                            w742 = 1  # 16 bit
                            w746 = 1  # Pos in Series
                            n181 = local read "Colormap"() -> (w743:u16)
                            n182 = case shown="0, Default" w743 {
                              tunnel: ["C:\\Users\\e14user\\Documents\\LabVIEW software\\GitRepo\\config\\Palettes\\Grey.pal" "C:\\Users\\e14user\\Documents\\LabVIEW software\\GitRepo\\config\\Palettes\\Hot.pal"] -> w744
                              frame 0, Default {
                              }
                              frame 1 {
                              }
                            }
                            n183 = Concatenate Strings(w753, ".tif" ("string")) -> (w751:string)
                            n184 = Build Path(base path=w754, name or relative path=w751) -> (appended path=w750:path)
                            n185 = Path To String(path=w750) -> (string=w745:string)
                            n186 = call <userlib>:"Save As Tiff.vi"("typ"=w742, "position"=w746, "palette"=w744, "path"=w745) -> ("function return"=w747:u32)  [unwired: 5 in, 2 out]
                            n187 = call "ConvertErrCodeToMessage.vi"("function return"=w747, "Array"=w749) -> ("Element Return"=w748:cluster{i32, string})  [unwired: 8 in, 1 out]
                          }
                          frame 7 {
                            n188 = local read "Colormap"() -> (w759:u16)
                            n189 = case shown="0, Default" w759 {
                              tunnel: ["C:\\Users\\e14user\\Documents\\LabVIEW software\\GitRepo\\config\\Palettes\\Grey.pal" "C:\\Users\\e14user\\Documents\\LabVIEW software\\GitRepo\\config\\Palettes\\Hot.pal"] -> w757
                              frame 0, Default {
                              }
                              frame 1 {
                              }
                            }
                            n190 = call <userlib>:"Save To Clip Board.vi"("palette"=w757) -> ("function return"=w758:u32)  [unwired: 8 in, 2 out]
                            n191 = call "ConvertErrCodeToMessage.vi"("function return"=w758) -> ("Element Return"=w760:cluster{i32, string})  [unwired: 9 in, 1 out]
                          }
                        }
                      }
                      frame #4 {
                        n192 = Build Array(w765, w764) -> (w763:cluster{i32, string}[])
                        n193 = local write "Acq. Error Array"(w763) -> ()
                      }
                    }
                  }
                  frame True {
                  }
                }
                n194 = local write "Save Image"(FALSE ("Save Image")) -> ()
              }
              event "Exposure": Value Change {
                n195 = event-data() -> ("NewVal"=w766:sgl)  [unwired: 1 in, 5 out]
                n196 = flat-sequence {
                  tunnel: [w769] -> w767
                  tunnel: w766 -> [w770]
                  tunnel: w767 -> [w779]
                  frame #0 {
                    n197 = while {
                      tunnel: w770 -> [w771]
                      tunnel: [w771] -> w769
                      stop <- w772 stop-if-true
                      n198 = call "Get Status.vi"() -> ("function return"=w778:u32, "status out"=w775:i32)  [unwired: 10 in]
                      n199 = Equal?(x=20073 ("status out"), y=w775) -> (x = y?=w774:bool)
                      n200 = Equal?(x=w778, y=20002 ("x")) -> (x = y?=w773:bool)
                      n201 = And(x=w774, y=w773) -> (x .and. y?=w772:bool)
                    }
                  }
                  frame #1 {
                    n202 = Divide(x=w779, y=sgl 1000.0) -> (x/y=w781:sgl)
                    n203 = call "Set Exposure Time.vi"("time"=w781) -> ()  [unwired: 10 in, 1 out]
                  }
                }
              }
              event "Single Image": Value Change {
                n204 = event-data() -> ("NewVal"=w786:bool)  [unwired: 1 in, 5 out]
                n205 = flat-sequence {
                  tunnel: w786 -> [w791]
                  tunnel: [w791] -> w782
                  tunnel: [w795] -> w783
                  tunnel: w782 -> [w795]
                  tunnel: w785 -> [w796]
                  tunnel: w783 -> [w797]
                  frame #0 {
                    w789 = 1  # Single Scan
                    w790 = 4  # Image Read
                    n206 = call "Set Number Accumulations.vi"("number"=1) -> ()  [unwired: 10 in, 1 out]
                    n207 = call "Set Number Kinetics.vi"("number"=1) -> ()  [unwired: 10 in, 1 out]
                    n208 = call "Set Acquisition Mode.vi"("mode"=w789) -> ()  [unwired: 10 in, 1 out]
                    n209 = call "Set Read Mode.vi"("mode"=w790) -> ()  [unwired: 10 in, 1 out]
                  }
                  frame #1 {
                    n210 = local read "Exposure"() -> (w792:sgl)
                    n211 = Divide(x=w792, y=sgl 1000.0) -> (x/y=w794:sgl)
                    n212 = call "Set Exposure Time.vi"("time"=w794) -> ()  [unwired: 10 in, 1 out]
                  }
                  frame #2 {
                    n213 = case shown="True" w797 {
                      tunnel: w796 -> [_ w807]
                      frame False {
                      }
                      frame True {
                        n214 = flat-sequence {
                          tunnel: w807 -> [w808]
                          tunnel: [w810] -> w806
                          tunnel: [w809] -> w805
                          tunnel: w806 -> [w812]
                          tunnel: w805 -> [w813]
                          tunnel: [w813] -> w804
                          tunnel: [w812] -> w803
                          tunnel: w804 -> [w828]
                          tunnel: w803 -> [w827]
                          tunnel: [w828] -> w802
                          tunnel: [w827] -> w801
                          tunnel: [w823] -> w800
                          tunnel: [w824] -> w799
                          tunnel: w802 -> [w832]
                          tunnel: w801 -> [w830]
                          tunnel: w800 -> [w831]
                          tunnel: w799 -> [w834]
                          tunnel: [w834] -> w798
                          tunnel: w798 -> [w846]
                          frame #0 {
                            n215 = call "Start Acquisition.vi"() -> ("function return"=w811:u32)  [unwired: 11 in]
                            n216 = call "ConvertErrCodeToMessage.vi"("function return"=w811, "Array"=w808) -> ("Element Return"=w809:cluster{i32, string}, "Array out"=w810:cluster{i32, string}[])  [unwired: 8 in]
                          }
                          frame #1 {
                            n217 = while {
                              stop <- w814 stop-if-true
                              n218 = call "Get Status.vi"() -> ("function return"=w820:u32, "status out"=w817:i32)  [unwired: 10 in]
                              n219 = Equal?(x=w820, y=20002 ("x")) -> (x = y?=w815:bool)
                              n220 = Equal?(x=20073 ("status out"), y=w817) -> (x = y?=w816:bool)
                              n221 = And(x=w816, y=w815) -> (x .and. y?=w814:bool)
                            }
                          }
                          frame #2 {
                            n222 = Square(x=1024) -> (x^2=w821:i32)
                            n223 = Initialize Array(i16 0 ("element"), w821) -> (w822:i16[])
                            n224 = call <userlib>:"Get Most Recent Image16.vi"("size"=w821, "arr"=w822) -> ("function return"=w823:u32, "arr out"=w824:u16[])  [unwired: 7 in, 1 out]
                          }
                          frame #3 {
                            n225 = call "ConvertErrCodeToMessage.vi"("function return"=w831, "Array"=w830) -> ("Element Return"=w833:cluster{i32, string})  [unwired: 8 in, 1 out]
                            n226 = Build Array(w833, w832) -> (w829:cluster{i32, string}[])
                            n227 = local write "Acq. Error Array"(w829) -> ()
                          }
                          frame #4 {
                            w849 = u32 2 items=["Zero Order", "Bi-Linear", "Quadratic", "Cubic Spline"] ("Interpolation Type")
                            w848 = T11 1 items=["Grayscale (U8)", "Grayscale (I16)", "Grayscale (SGL)", "Complex (CSG)", "RGB (U32)", "HSL (U32)", "RGB (U64)", "Grayscale (U16)"] ("Image Type")
                            w847 = 1024 ("dimension size")
                            n228 = local read "Image Name"() -> (w845:string)
                            n229 = Reshape Array(w846, w847, w847) -> (w851:u16[][])
                            n230 = call "IMAQ Create"("Image Name"=w845, "Image Type"=w848) -> ("New Image"=w850:T8)  [unwired: 3 in, 1 out]
                            n231 = property on="Image" class="ImageControl"() -> ("Image Area Height"=w842:u32, "Image Area Width"=w843:u32)  [unwired: 2 in, 2 out]
                            n232 = call "IMAQ ArrayToImage"("Image Pixels (I16)"=w851, "Image"=w850) -> ("Image Out"=w844:T8)  [unwired: 8 in, 1 out]
                            n233 = call "IMAQ GetImageSize"("Image"=w844) -> ("Y Resolution"=w836:i32, "X Resolution"=w839:i32)  [unwired: 3 in, 1 out]
                            n234 = Divide(x=w836, y=w842) -> (x/y=w852:dbl)
                            n235 = Divide(x=w839, y=w843) -> (x/y=w853:dbl)
                            n236 = Max & Min(x=w852, y=w853) -> (max(x,y)=w841:dbl, min(x,y)=w837:dbl)
                            n237 = Divide(x=w839, y=w841) -> (x/y=w840:dbl)
                            n238 = Divide(x=w836, y=w837) -> (x/y=w838:dbl)
                            n239 = call "IMAQ Resample"("X Resolution"=w840, "Y Resolution"=w838, "Interpolation Type"=w849, "Image Src"=w844) -> ("Image Dst Out"=w835:T8)  [unwired: 6 in, 1 out]
                            n240 = local write "Image"(w835) -> ()
                          }
                          frame #5 {
                            n241 = local write "Single Image"(FALSE ("Single Image")) -> ()
                          }
                        }
                      }
                    }
                  }
                }
              }
              event "Live Mode": Value Change {
                n242 = event-data() -> ("NewVal"=w855:bool)  [unwired: 1 in, 5 out]
              }
            }
            n243 = case shown="False" w640 {
              selector: w640 -> [w856 _]
              tunnel: [w856 FALSE] -> w638
              frame False {
              }
              frame True {
                n244 = flat-sequence {
                  frame #0 {
                    n245 = property on="Exposure" class="DigNum (strict)"("DisabledEnum"=T9."Disabled and Grayed Out" ("Disabled")) -> ()  [unwired: 2 in, 2 out]
                  }
                  frame #1 {
                    w859 = 4  # Image
                    n246 = call "Set Read Mode.vi"("mode"=w859) -> ()  [unwired: 10 in, 1 out]
                  }
                  frame #2 {
                    n247 = call "Set Kinetic Cycle Time.vi"("time"=sgl 0.0) -> ()  [unwired: 10 in, 1 out]
                  }
                  frame #3 {
                    w861 = 5  # Run till abort
                    n248 = call "Set Acquisition Mode.vi"("mode"=w861) -> ()  [unwired: 10 in, 1 out]
                  }
                  frame #4 {
                    n249 = call "Start Acquisition.vi"() -> ()  [unwired: 11 in, 1 out]
                  }
                  frame #5 {
                    n250 = while {
                      stop <- w865 stop-if-true
                      # "Live Mode Loop"
                      n251 = case shown="\"\", Default" "" {
                        frame "", Default {
                          n252 = local read "Image Name"() -> (w867:string)
                          n253 = call "AndorLiveMode.vi"("Image Name"=w867) -> ("Image"=w868:T8)  [unwired: 9 in, 1 out]
                          n254 = local write "Image"(w868) -> ()
                        }
                        frame "Exposure" {
                          n255 = stacked-sequence {
                            frame #0 {
                              n256 = call "Abort Acquisition.vi"() -> ()  [unwired: 11 in, 1 out]
                            }
                            frame #1 {
                              n257 = while {
                                stop <- w869 stop-if-true
                                n258 = call "Get Status.vi"() -> ("function return"=w875:u32, "status out"=w872:i32)  [unwired: 10 in]
                                n259 = Equal?(x=20073 ("status out"), y=w872) -> (x = y?=w871:bool)
                                n260 = Equal?(x=w875, y=20002 ("x")) -> (x = y?=w870:bool)
                                n261 = And(x=w871, y=w870) -> (x .and. y?=w869:bool)
                              }
                            }
                            frame #2 {
                              n262 = local read "Exposure"() -> (w878:sgl)
                              n263 = Divide(x=w878, y=sgl 1000.0) -> (x/y=w877:sgl)
                              n264 = call "Set Exposure Time.vi"("time"=w877) -> ()  [unwired: 10 in, 1 out]
                            }
                            frame #3 {
                              n265 = call "Start Acquisition.vi"() -> ()  [unwired: 11 in, 1 out]
                            }
                          }
                        }
                      }
                      n266 = local read "Live Mode"() -> (w864:bool)
                      n267 = local read "stop"() -> (w863:bool)
                      n268 = Not(x=w864) -> (.not. x?=w862:bool)
                      n269 = Or(x=w863, y=w862) -> (x .or. y?=w865:bool)
                    }
                  }
                  frame #6 {
                    n270 = call "Abort Acquisition.vi"() -> ()  [unwired: 11 in, 1 out]
                  }
                  frame #7 {
                    n271 = local write "Live Mode"(FALSE ("Live Mode")) -> ()
                    n272 = property on="Exposure" class="DigNum (strict)"("DisabledEnum"=T9."Enabled" ("Disabled")) -> ()  [unwired: 2 in, 2 out]
                  }
                }
              }
            }
            n273 = event shown="[0] Timeout" {
              selector: _ -> [_]
              dyn-events: _ -> [_]
              timeout: 2000 -> [_]
              event Timeout {
                n274 = event-data() -> ()  [unwired: 1 in, 3 out]
                n275 = call "Get Temperature F.vi"() -> ("temperature out"=w642:sgl)  [unwired: 10 in, 1 out]
                n276 = local write "Camera Temperature"(w642) -> ()
              }
            }
            n277 = local read "stop"() -> (w635:bool)
          }
        }
      }
      n278 = local read "LINX Resource"() -> (w223:T1)
      n279 = local read "TANGO ID"() -> (w234:i32)
      n280 = Obtain Queue(name (unnamed)="FluidCTRL", element data type=w229, error in (no error)=w228) -> (queue out=w224:refnum<queue>, error out=w225:errorcluster)  [unwired: 2 in, 1 out]
      n281 = Obtain Queue(name (unnamed)="StageCTRL", element data type=w239, error in (no error)=w228) -> (queue out=w235:refnum<queue>, error out=w236:errorcluster)  [unwired: 2 in, 1 out]
      n282 = while {
        tunnel: w235 -> [w547]
        tunnel: w236 -> [w546]
        tunnel: [w551] -> w238
        tunnel: [w548] -> w237
        stop <- w550 stop-if-true
        # "TANGO Stage Message Loop"
        n283 = event shown="[8] \"Export List\": Value Change" {
          selector: _ -> [_ _ _ _ _ _ _ _ _]
          dyn-events: _ -> [_ _ _ _ _ _ _ _ _]
          timeout: 0 -> [_ _ _ _ _ _ _ _ _]
          tunnel: w546 -> [w554 w557 w563 w574 w582 w587 w599 w611 w621]
          tunnel: [w554 w558 w566 w573 w581 w589 w601 w614 w623] -> w548
          tunnel: [w553 w559 w565 w572 w580 w590 w602 w615 w624] -> w551
          tunnel: w547 -> [w553 w556 w564 w575 w579 w588 w600 w612 w622]
          event Timeout {
            n284 = event-data() -> ()  [unwired: 1 in, 3 out]
          }
          event "Up": Value Change {
            n285 = event-data() -> ("NewVal"=w555:bool)  [unwired: 1 in, 5 out]
            n286 = case shown="False" w555 {
              tunnel: ["UP RELEASED" "UP PRESSED"] -> w560
              frame False {
              }
              frame True {
              }
            }
            n287 = Enqueue Element(queue=w556, element=w560, error in (no error)=w557) -> (queue out=w559:refnum<queue>, error out=w558:errorcluster)  [unwired: 1 in, 1 out]
          }
          event "Down": Value Change {
            n288 = event-data() -> ("NewVal"=w567:bool)  [unwired: 1 in, 5 out]
            n289 = case shown="True" w567 {
              tunnel: ["DOWN RELEASED" "DOWN PRESSED"] -> w568
              frame False {
              }
              frame True {
              }
            }
            n290 = Enqueue Element(queue=w564, element=w568, error in (no error)=w563) -> (queue out=w565:refnum<queue>, error out=w566:errorcluster)  [unwired: 1 in, 1 out]
          }
          event "Left": Value Change {
            n291 = event-data() -> ("NewVal"=w571:bool)  [unwired: 1 in, 5 out]
            n292 = case shown="False" w571 {
              tunnel: ["LEFT RELEASED" "LEFT PRESSED"] -> w576
              frame False {
              }
              frame True {
              }
            }
            n293 = Enqueue Element(queue=w575, element=w576, error in (no error)=w574) -> (queue out=w572:refnum<queue>, error out=w573:errorcluster)  [unwired: 1 in, 1 out]
          }
          event "Right": Value Change {
            n294 = event-data() -> ("NewVal"=w584:bool)  [unwired: 1 in, 5 out]
            n295 = case shown="True" w584 {
              tunnel: ["RIGHT RELEASED" "RIGHT PRESSED"] -> w583
              frame False {
              }
              frame True {
              }
            }
            n296 = Enqueue Element(queue=w579, element=w583, error in (no error)=w582) -> (queue out=w580:refnum<queue>, error out=w581:errorcluster)  [unwired: 1 in, 1 out]
          }
          event "Save Pos": Value Change {
            n297 = event-data() -> ("NewVal"=w591:bool)  [unwired: 1 in, 5 out]
            n298 = case shown="True" w591 {
              tunnel: [w595 w597] -> w590
              tunnel: [w594 w598] -> w589
              tunnel: w588 -> [w593 w597]
              tunnel: w587 -> [w592 w598]
              frame True {
                n299 = Enqueue Element(queue=w593, element="SAVEPOS", error in (no error)=w592) -> (queue out=w595:refnum<queue>, error out=w594:errorcluster)  [unwired: 1 in, 1 out]
              }
              frame False {
              }
            }
          }
          event "Clear Last Pos": Value Change {
            n300 = event-data() -> ("NewVal"=w603:bool)  [unwired: 1 in, 5 out]
            n301 = case shown="True" w603 {
              tunnel: [w607 w609] -> w602
              tunnel: [w606 w610] -> w601
              tunnel: w600 -> [w605 w609]
              tunnel: w599 -> [w604 w610]
              frame True {
                n302 = Enqueue Element(queue=w605, element="CLEARPOS", error in (no error)=w604) -> (queue out=w607:refnum<queue>, error out=w606:errorcluster)  [unwired: 1 in, 1 out]
              }
              frame False {
              }
            }
          }
          event "Position List": Value Change {
            n303 = event-data() -> ("NewVal"=w619:i32[])  [unwired: 1 in, 5 out]
            n304 = Number To Decimal String(number=w619) -> (decimal integer string=w617:string[])  [unwired: 1 in]
            n305 = call <vilib>:"Space Constant.vi"() -> ("String"=w618:string)
            n306 = Concatenate Strings("SELECTPOS", w618, w617) -> (w613:string)
            n307 = Enqueue Element(queue=w612, element=w613, error in (no error)=w611) -> (queue out=w615:refnum<queue>, error out=w614:errorcluster)  [unwired: 1 in, 1 out]
          }
          event "Export List": Value Change {
            n308 = event-data() -> ("NewVal"=w620:bool)  [unwired: 1 in, 5 out]
            n309 = case shown="False" w620 {
              tunnel: [w626 w631] -> w624
              tunnel: [w625 w630] -> w623
              tunnel: w622 -> [w626 w629]
              tunnel: w621 -> [w625 w628]
              frame False {
              }
              frame True {
                n310 = Enqueue Element(queue=w629, element="EXPORT", error in (no error)=w628) -> (queue out=w631:refnum<queue>, error out=w630:errorcluster)  [unwired: 1 in, 1 out]
              }
            }
          }
        }
        n311 = local read "stop"() -> (w549:bool)
        n312 = Or(x=w548, y=w549) -> (x .or. y?=w550:bool)
      }
      n313 = while {
        tunnel: w224 -> [w283]
        tunnel: w225 -> [w282]
        tunnel: [w287] -> w227
        tunnel: [w284] -> w226
        stop <- w286 stop-if-true
        # "Fluid Message Handling Loop"
        n314 = event shown="[0] Timeout" {
          selector: _ -> [_ _ _ _]
          dyn-events: _ -> [_ _ _ _]
          timeout: 0 -> [_ _ _ _]
          tunnel: w282 -> [w290 w292 w304 w316]
          tunnel: [w290 w295 w307 w319] -> w287
          tunnel: [w289 w294 w306 w318] -> w284
          tunnel: w283 -> [w289 w293 w305 w317]
          event Timeout {
            n315 = event-data() -> ()  [unwired: 1 in, 3 out]
          }
          event "Feed On": Value Change {
            n316 = event-data() -> ("NewVal"=w291:bool)  [unwired: 1 in, 5 out]
            n317 = case shown="False" w291 {
              tunnel: [w296 w302] -> w295
              tunnel: [w297 w301] -> w294
              tunnel: w293 -> [w297 w300]
              tunnel: w292 -> [w296 w299]
              frame False {
              }
              frame True {
                n318 = Enqueue Element(queue=w300, element="FEED", error in (no error)=w299) -> (queue out=w301:refnum<queue>, error out=w302:errorcluster)  [unwired: 1 in, 1 out]
              }
            }
          }
          event "Pump On": Value Change {
            n319 = event-data() -> ("NewVal"=w303:bool)  [unwired: 1 in, 5 out]
            n320 = case shown="True" w303 {
              tunnel: [w308 w314] -> w307
              tunnel: [w309 w313] -> w306
              tunnel: w305 -> [w309 w312]
              tunnel: w304 -> [w308 w311]
              frame False {
              }
              frame True {
                n321 = Enqueue Element(queue=w312, element="PUMP", error in (no error)=w311) -> (queue out=w313:refnum<queue>, error out=w314:errorcluster)  [unwired: 1 in, 1 out]
              }
            }
          }
          event "Flush": Value Change {
            n322 = event-data() -> ("NewVal"=w315:bool)  [unwired: 1 in, 5 out]
            n323 = case shown="False" w315 {
              tunnel: [w324 w329] -> w319
              tunnel: [w323 w328] -> w318
              tunnel: w317 -> [w322 w327]
              tunnel: w316 -> [w321 w326]
              frame True {
                n324 = Enqueue Element(queue=w322, element="FLUSH ON", error in (no error)=w321) -> (queue out=w323:refnum<queue>, error out=w324:errorcluster)  [unwired: 1 in, 1 out]
              }
              frame False, Default {
                n325 = Enqueue Element(queue=w327, element="FLUSH OFF", error in (no error)=w326) -> (queue out=w328:refnum<queue>, error out=w329:errorcluster)  [unwired: 1 in, 1 out]
              }
            }
          }
        }
        n326 = local read "stop"() -> (w285:bool)
        n327 = Or(x=w287, y=w285) -> (x .or. y?=w286:bool)
      }
      n328 = while {
        tunnel: w224 -> [w251]
        shift-right: [w246] -> _
        shift-left: w225 -> [w250]
        tunnel: w223 -> [w247]
        stop <- w246 stop-if-true
        n329 = Dequeue Element(queue=w251, error in (no error)=w250) -> (element=w249:string, error out=w248:errorcluster)  [unwired: 1 in, 2 out]
        n330 = case shown="\"FLUSH OFF\"" w249 {
          tunnel: w248 -> [w258 w269 w275 w281]
          tunnel: [w255 w264 w271 w277] -> w246
          tunnel: w247 -> [w252 w266 w274 w280]
          frame "FEED" {
            n331 = local read "Feed\nReagent"() -> (w257:u16)
            n332 = local read "Ring"() -> (w260:u16)
            n333 = local read "Feed Cycles"() -> (w259:i32)
            n334 = local read "Single/\nMultiring?"() -> (w261:bool)
            n335 = local read "All Rings"() -> (w256:bool)
            n336 = call "ArdnoFeed.vi"("LINX Resource"=w252, "Single / Multivalve?"=w261, "Channel"=w257, "Ring"=w260, "Feed Cycles"=w259, "error in (no error)"=w258, "All Rings"=w256) -> ("error out"=w254:errorcluster)  [unwired: 7 in, 1 out]
            n337 = property on="Feed On" class="Bool (strict)"(error in=w254, "Value"=FALSE ("Feed On")) -> (error out=w255:errorcluster)  [unwired: 1 in, 1 out]
          }
          frame "PUMP" {
            n338 = local read "Frequency"() -> (w268:dbl)
            n339 = local read "Pump Cycles"() -> (w267:dbl)
            n340 = local read "Single/\nMultiring?"() -> (w265:bool)
            n341 = call "ArdnoPump.vi"("LINX Resource"=w266, "Pump Cycles"=w267, "Pump Frequency"=w268, "error in (no error)"=w269, "Single/\nMultiring?"=w265) -> ("error out"=w263:errorcluster)  [unwired: 1 out]
            n342 = property on="Pump On" class="Bool (strict)"(error in=w263, "Value"=FALSE ("Pump On")) -> (error out=w264:errorcluster)  [unwired: 1 in, 1 out]
          }
          frame "FLUSH ON", Default {
            n343 = local read "Single/\nMultiring?"() -> (w272:bool)
            n344 = local read "Flush\nReagent"() -> (w273:u16)
            n345 = call "ArdnoFlush.vi"("Open?"=FALSE, "error in (no error)"=w275, "Single / Multivalve?"=w272, "Channel"=w273, "LINX Resource"=w274) -> ("error out"=w271:errorcluster)  [unwired: 5 in, 1 out]
          }
          frame "FLUSH OFF" {
            n346 = local read "Single/\nMultiring?"() -> (w278:bool)
            n347 = local read "Flush\nReagent"() -> (w279:u16)
            n348 = call "ArdnoFlush.vi"("Open?"=TRUE, "error in (no error)"=w281, "Single / Multivalve?"=w278, "Channel"=w279, "LINX Resource"=w280) -> ("error out"=w277:errorcluster)  [unwired: 5 in, 1 out]
          }
        }
      }
      n349 = while {
        tunnel: w235 -> [w339]
        tunnel: w234 -> [w334]
        shift-right: [w330] -> _
        shift-left: w236 -> [w338]
        stop <- w330 stop-if-true
        # "TANGO Stage Execution Loop"
        n350 = Dequeue Element(queue=w339, error in (no error)=w338) -> (element=w332:string, error out=w333:errorcluster)  [unwired: 1 in, 2 out]
        n351 = call <vilib>:"Space Constant.vi"() -> ("String"=w337:string)
        n352 = Match Pattern(string=w332, regular expression=w337) -> (before substring=w336:string, after substring=w335:string)  [unwired: 1 in, 2 out]
        n353 = case shown="\"SELECTPOS\"" w336 {
          tunnel: w335 -> [w344 w368 w392 w416 _ _ w537 _]
          tunnel: w334 -> [w343 w367 w391 w415 w477 _ w526 _]
          tunnel: w333 -> [w342 w366 w390 w414 w470 w481 w519 w540]
          tunnel: [w341 w365 w389 w413 w445 w481 w491 w539] -> w330
          tunnel: [w340 w364 w388 w412 FALSE FALSE FALSE FALSE] -> _
          frame "DOWN", Default {
            n354 = case shown="\"PRESSED\"" w344 {
              tunnel: w342 -> [w346 w363]
              tunnel: [w346 w362] -> w341
              tunnel: w343 -> [_ w351]
              tunnel: [FALSE TRUE] -> w340
              frame "RELEASED", Default {
              }
              frame "PRESSED" {
                n355 = local read "TangoStep"() -> (w349:dbl)
                n356 = Multiply(x=1.0, y=w349) -> (x*y=w352:dbl)
                n357 = call <userlib>:"LSX Move Rel.vi"("bWait"=0.0, "dA"=0.0, "dZ"=0.0, "error in (no error)"=w363, "dY"=w352, "dX"=0.0 ("dY"), "lLSID"=w351) -> ("error out"=w354:errorcluster)  [unwired: 3 in, 1 out]
                n358 = call <userlib>:"LSX Get Pos.vi"("lLSID"=w351, "error in (no error)"=w354) -> ("pdA out"=w355:dbl, "pdX out"=w358:dbl, "pdY out"=w357:dbl, "pdZ out"=w356:dbl, "error out"=w362:errorcluster)  [unwired: 8 in, 1 out]
                n359 = Build Array(w358, w357, w356, w355) -> (w348:dbl[])
                n360 = local write "Position"(w348) -> ()
              }
            }
          }
          frame "UP" {
            n361 = case shown="\"PRESSED\"" w368 {
              tunnel: w366 -> [w370 w387]
              tunnel: [w370 w386] -> w365
              tunnel: w367 -> [_ w375]
              tunnel: [FALSE TRUE] -> w364
              frame "RELEASED", Default {
              }
              frame "PRESSED" {
                n362 = local read "TangoStep"() -> (w373:dbl)
                n363 = Multiply(x=-1.0, y=w373) -> (x*y=w376:dbl)
                n364 = call <userlib>:"LSX Move Rel.vi"("bWait"=0.0, "dA"=0.0, "dZ"=0.0, "error in (no error)"=w387, "dY"=w376, "dX"=0.0 ("dY"), "lLSID"=w375) -> ("error out"=w378:errorcluster)  [unwired: 3 in, 1 out]
                n365 = call <userlib>:"LSX Get Pos.vi"("lLSID"=w375, "error in (no error)"=w378) -> ("pdA out"=w379:dbl, "pdX out"=w382:dbl, "pdY out"=w381:dbl, "pdZ out"=w380:dbl, "error out"=w386:errorcluster)  [unwired: 8 in, 1 out]
                n366 = Build Array(w382, w381, w380, w379) -> (w372:dbl[])
                n367 = local write "Position"(w372) -> ()
              }
            }
          }
          frame "LEFT" {
            n368 = case shown="\"PRESSED\"" w392 {
              tunnel: w390 -> [w394 w411]
              tunnel: [w394 w410] -> w389
              tunnel: w391 -> [_ w400]
              tunnel: [FALSE TRUE] -> w388
              frame "RELEASED", Default {
              }
              frame "PRESSED" {
                n369 = local read "TangoStep"() -> (w399:dbl)
                n370 = Multiply(x=-1.0, y=w399) -> (x*y=w395:dbl)
                n371 = call <userlib>:"LSX Move Rel.vi"("bWait"=0.0, "dA"=0.0, "dZ"=0.0, "error in (no error)"=w411, "dY"=0.0, "dX"=w395, "lLSID"=w400) -> ("error out"=w402:errorcluster)  [unwired: 3 in, 1 out]
                n372 = call <userlib>:"LSX Get Pos.vi"("lLSID"=w400, "error in (no error)"=w402) -> ("pdA out"=w403:dbl, "pdX out"=w406:dbl, "pdY out"=w405:dbl, "pdZ out"=w404:dbl, "error out"=w410:errorcluster)  [unwired: 8 in, 1 out]
                n373 = Build Array(w406, w405, w404, w403) -> (w398:dbl[])
                n374 = local write "Position"(w398) -> ()
              }
            }
          }
          frame "RIGHT" {
            n375 = case shown="\"PRESSED\"" w416 {
              tunnel: w414 -> [w418 w435]
              tunnel: [w418 w434] -> w413
              tunnel: w415 -> [_ w424]
              tunnel: [FALSE TRUE] -> w412
              frame "RELEASED", Default {
              }
              frame "PRESSED" {
                n376 = local read "TangoStep"() -> (w423:dbl)
                n377 = Multiply(x=1.0, y=w423) -> (x*y=w419:dbl)
                n378 = call <userlib>:"LSX Move Rel.vi"("bWait"=0.0, "dA"=0.0, "dZ"=0.0, "error in (no error)"=w435, "dY"=0.0, "dX"=w419, "lLSID"=w424) -> ("error out"=w426:errorcluster)  [unwired: 3 in, 1 out]
                n379 = call <userlib>:"LSX Get Pos.vi"("lLSID"=w424, "error in (no error)"=w426) -> ("pdA out"=w427:dbl, "pdX out"=w430:dbl, "pdY out"=w429:dbl, "pdZ out"=w428:dbl, "error out"=w434:errorcluster)  [unwired: 8 in, 1 out]
                n380 = Build Array(w430, w429, w428, w427) -> (w422:dbl[])
                n381 = local write "Position"(w422) -> ()
              }
            }
          }
          frame "SAVEPOS" {
            n382 = local read "IX 81 Port"() -> (w469:refnum<visa-resource-name>)
            n383 = call <userlib>:"LSX Get Pos.vi"("lLSID"=w477, "error in (no error)"=w470) -> ("pdX out"=w475:dbl, "pdY out"=w474:dbl, "error out"=w448:errorcluster)  [unwired: 8 in, 3 out]
            n384 = call "OlympusQuery.vi"("error in (no error)"=w470, "Device Number\n(1: -Condensor\n     - Objective\n     - Lamp\n     - Shutter\n2: - Z-Motion\n   - Autofocus)"=2 ("Device Number\n(1: -Condensor\n     - Objective\n     - Lamp\n     - Shutter\n2: - Z-Motion\n   - Autofocus)"), "String"="POS?", "VISA Resource Name In"=w469) -> ("error out"=w461:errorcluster, "Result"=w462:string, "VISA Resource Name Out"=w439:refnum<visa-resource-name>)  [unwired: 5 in]
            n385 = Decimal String To Number(string=w462, default (0L)=0.0 ("default (0 I32)")) -> (number=w437:dbl)  [unwired: 1 in, 1 out]
            n386 = Divide(x=w437, y=1000.0) -> (x/y=w438:dbl)
            n387 = call "OlympusQuery.vi"("error in (no error)"=w461, "Device Number\n(1: -Condensor\n     - Objective\n     - Lamp\n     - Shutter\n2: - Z-Motion\n   - Autofocus)"=1 ("Device Number\n(1: -Condensor\n     - Objective\n     - Lamp\n     - Shutter\n2: - Z-Motion\n   - Autofocus)"), "String"="OB?", "VISA Resource Name In"=w439) -> ("error out"=w452:errorcluster, "Result"=w468:string, "VISA Resource Name Out"=w453:refnum<visa-resource-name>)  [unwired: 5 in]
            n388 = Decimal String To Number(string=w468) -> (number=w464:i32)  [unwired: 2 in, 1 out]
            n389 = property on="Objective" class="Enum (strict)"() -> ("Strings []"=w465:string[])  [unwired: 2 in, 2 out]
            n390 = Decrement(x=w464) -> (x-1=w463:i32)
            n391 = Index Array(array=w465, index=w463) -> (element=w460:string)
            n392 = call "OlympusQuery.vi"("error in (no error)"=w452, "Device Number\n(1: -Condensor\n     - Objective\n     - Lamp\n     - Shutter\n2: - Z-Motion\n   - Autofocus)"=1 ("Device Number\n(1: -Condensor\n     - Objective\n     - Lamp\n     - Shutter\n2: - Z-Motion\n   - Autofocus)"), "String"="MU?", "VISA Resource Name In"=w453) -> ("error out"=w449:errorcluster, "Result"=w459:string)  [unwired: 5 in, 1 out]
            n393 = property on="Filter" class="Ring (strict)"() -> ("Strings []"=w454:string[])  [unwired: 2 in, 2 out]
            n394 = Decimal String To Number(string=w459) -> (number=w456:i32)  [unwired: 2 in, 1 out]
            n395 = Decrement(x=w456) -> (x-1=w455:i32)
            n396 = Index Array(array=w454, index=w455) -> (element=w451:string)
            n397 = local read "Intensity [%]"() -> (w450:dbl)
            n398 = local write "Save Pos"(FALSE ("Save Pos")) -> ()
            n399 = Bundle("pdX out"=w475, "pdY out"=w474, w438, w460, w451, "Intensity [%]"=w450) -> (w443:T12)  [unwired: 1 in]
            n400 = Merge Errors(w448, w449) -> (w446:errorcluster)
            n401 = property on="Position List" class="MCListbox (strict)"() -> ("ItemNames"=w442:string[][])  [unwired: 2 in, 2 out]
            n402 = Build Array(w443) -> (w444:T13)
            n403 = call "TangoPositions2MultiList.vi"("error in (no error)"=w446, "Saved Positions"=w444) -> ("error out"=w445:errorcluster, "Array"=w441:string[][])  [unwired: 8 in]
            n404 = Build Array (concatenate)(w442, w441) -> (w440:string[][])
            n405 = property on="Position List" class="MCListbox (strict)"("ItemNames"=w440) -> ()  [unwired: 2 in, 2 out]
          }
          frame "CLEARPOS" {
            n406 = property on="Position List" class="MCListbox (strict)"() -> ("ItemNames"=w485:string[][])  [unwired: 2 in, 2 out]
            n407 = Array Size(array=w485) -> (size(s)=w483:i32[])
            n408 = Index Array(array=w483, index=0) -> (element=w482:i32)
            n409 = Decrement(x=w482) -> (x-1=w486:i32)
            n410 = Delete From Array(array=w485, index (row)=w486) -> (array with subset deleted=w478:string[][])  [unwired: 2 in, 1 out]
            n411 = property on="Position List" class="MCListbox (strict)"("ItemNames"=w478) -> ()  [unwired: 2 in, 2 out]
            n412 = local write "Clear Last Pos"(FALSE ("Clear Last Pos")) -> ()
          }
          frame "SELECTPOS" {
            w527 = 0.0
            n413 = property on="Position List" class="MCListbox (strict)"() -> ("ItemNames"=w538:string[][])  [unwired: 2 in, 2 out]
            n414 = Decimal String To Number(string=w537) -> (number=w536:i32)  [unwired: 2 in, 1 out]
            n415 = Index Array(array=w538, index (row)=w536) -> (element=w529:string[])  [unwired: 1 in]
            n416 = Index String Array(1:0 ("index"), 2:w529) -> (0:w528:string)  [unwired: 1 in]
            n417 = Index String Array(1:1 ("index"), 2:w529) -> (0:w524:string)  [unwired: 1 in]
            n418 = Decimal String To Number(string=w528, default (0L)=w527) -> (number=w525:dbl)  [unwired: 1 in, 1 out]
            n419 = Decimal String To Number(string=w524, default (0L)=w527) -> (number=w523:dbl)  [unwired: 1 in, 1 out]
            n420 = call <userlib>:"LSX Move Abs.vi"("error in (no error)"=w519, "dY"=w523, "dX"=w525, "lLSID"=w526) -> ()  [unwired: 6 in, 2 out]
            n421 = Index String Array(1:2 ("index"), 2:w529) -> (0:w522:string)  [unwired: 1 in]
            n422 = Decimal String To Number(string=w522, default (0L)=0.0 ("default (0 I32)")) -> (number=w518:dbl)  [unwired: 1 in, 1 out]
            n423 = Obtain Queue(name (unnamed)="MicroscopeCTRL", element data type=cluster{"Button":string, "Value":dbl} {"Button"="", "Value"=0.0}, error in (no error)=w519) -> (queue out=w516:refnum<queue>, error out=w515:errorcluster)  [unwired: 2 in, 1 out]
            n424 = Bundle("FOCUS", w518) -> (w517:cluster{string, dbl})  [unwired: 1 in]
            n425 = Enqueue Element(queue=w516, element=w517, error in (no error)=w515) -> (queue out=w507:refnum<queue>, error out=w508:errorcluster)  [unwired: 1 in, 1 out]
            n426 = property on="Objective" class="Enum (strict)"() -> ("Strings []"=w512:string[])  [unwired: 2 in, 2 out]
            n427 = Index String Array(1:3 ("index"), 2:w529) -> (0:w511:string)  [unwired: 1 in]
            n428 = Match First String(2:w512, 3:w511) -> (0:w504:i32)  [unwired: 1 out]
            n429 = Bundle("OBJECTIVE", "index"=w504) -> (w509:cluster{string, "index":i32})  [unwired: 1 in]
            n430 = Enqueue Element(queue=w507, element=w509, error in (no error)=w508) -> (queue out=w500:refnum<queue>, error out=w499:errorcluster)  [unwired: 1 in, 1 out]
            n431 = property on="Filter" class="Ring (strict)"() -> ("Strings []"=w505:string[])  [unwired: 2 in, 2 out]
            n432 = Index String Array(1:5 ("index"), 2:w529) -> (0:w506:string)  [unwired: 1 in]
            n433 = Match First String(2:w505, 3:w506) -> (0:w503:i32)  [unwired: 1 out]
            n434 = Increment(x=w503) -> (x+1=w487:i32)
            n435 = Bundle("FILTER", w487) -> (w501:cluster{string, i32})  [unwired: 1 in]
            n436 = Enqueue Element(queue=w500, element=w501, error in (no error)=w499) -> (queue out=w493:refnum<queue>, error out=w492:errorcluster)  [unwired: 1 in, 1 out]
            n437 = Index String Array(1:4 ("index"), 2:w529) -> (0:w498:string)  [unwired: 1 in]
            n438 = Decimal String To Number(string=w498, default (0L)=0.0 ("default (0 I32)")) -> (number=w496:dbl)  [unwired: 1 in, 1 out]
            n439 = Bundle("INTENSITY", w496) -> (w494:cluster{string, dbl})  [unwired: 1 in]
            n440 = Enqueue Element(queue=w493, element=w494, error in (no error)=w492) -> (queue out=w490:refnum<queue>, error out=w489:errorcluster)  [unwired: 1 in, 1 out]
            n441 = Release Queue(queue=w490, error in (no error)=w489) -> (error out=w491:errorcluster)  [unwired: 1 in, 2 out]
          }
          frame "EXPORT" {
            n442 = flat-sequence {
              tunnel: w540 -> [w544]
              tunnel: [w543] -> w539
              frame #0 {
                n443 = property on="Position List" class="MCListbox (strict)"() -> ("ItemNames"=w542:string[][])  [unwired: 2 in, 2 out]
                n444 = call "ExportPosList.vi"("error in (no error)"=w544, "Array"=w542) -> ("error out"=w543:errorcluster)  [unwired: 8 in, 1 out]
              }
              frame #1 {
                n445 = local write "Export List"(FALSE ("Export List")) -> ()
              }
            }
          }
        }
        n446 = Wait (ms)(milliseconds to wait=u32 50) -> ()  [unwired: 1 out]
      }
      n447 = Release Queue(queue=w226, error in (no error)=w227) -> (error out=w222:errorcluster)  [unwired: 1 in, 2 out]
      n448 = Release Queue(queue=w238, error in (no error)=w237) -> (error out=w232:errorcluster)  [unwired: 1 in, 2 out]
      n449 = local read "IX 81 Port"() -> (w241:refnum<visa-resource-name>)
      n450 = Obtain Queue(name (unnamed)="MicroscopeCTRL", element data type=cluster{"Button":string, "Value":dbl} {"Button"="", "Value"=0.0}, error in (no error)=w228) -> (queue out=w243:refnum<queue>, error out=w242:errorcluster)  [unwired: 2 in, 1 out]
      n451 = while {
        tunnel: w243 -> [w888]
        tunnel: [w887] -> _
        shift-right: [w882] -> _
        shift-left: w242 -> [w889]
        tunnel: w241 -> [w881]
        stop <- w882 stop-if-true
        # "Microsocope Actuation Loop"
        n452 = Dequeue Element(queue=w888, error in (no error)=w889) -> (queue out=w887:refnum<queue>, element=w886:cluster{"Button":string, "Value":dbl}, error out=w883:errorcluster)  [unwired: 1 in, 1 out]
        n453 = Unbundle By Name(w886) -> ("Button"=w885:string, "Value"=w884:dbl)
        n454 = case shown="\"FOCUSUPDATE\"" w885 {
          tunnel: w884 -> [w892 w905 w930 w938 w961 _ _ w981 _ w991]
          tunnel: w883 -> [w898 w904 w933 w936 w964 w967 w975 w982 w984 w993]
          tunnel: [w897 w901 w923 w935 w965 _ w977 w983 w985 w987] -> w882
          tunnel: w881 -> [w899 w907 w934 w937 w960 w966 w976 w980 _ _]
          frame "BF ENABLE" {
            n455 = local read "Lamp Type (0: Transmitted)"() -> (w896:enum16{"Transmitted", "Reflected"})
            n456 = Not Equal To 0?(x=w892) -> (x != 0?=w893:bool)
            n457 = local read "Intensity [%]"() -> (w894:dbl)
            n458 = local write "Filter"(T10."BF (empty)" ("Filter")) -> ()
            n459 = Multiply(x=0.12, y=w894) -> (x*y=w891:dbl)
            n460 = call "Configure Lamp.vi"("VISA Resource Name"=w899, "Lamp Intensity (1.0 V)"=w891, "Lamp Enabled (True)"=w893, "Lamp Type (0: Transmitted)"=w896, "error in (no error)"=w898) -> ("error out"=w897:errorcluster)  [unwired: 9 in, 1 out]
          }
          frame "FILTER" {
            n461 = To Unsigned Long Integer(number=w905) -> (unsigned 32bit integer=w906:u32)
            n462 = Increment(x=w906) -> (x+1=w900:u32)
            n463 = call "Select Filter Wheel.vi"("error in (no error)"=w904, "Filter Wheel Position (1)"=w900, "VISA Resource Name"=w907) -> ("error out"=w903:errorcluster, "VISA Resource Name Out"=w902:refnum<visa-resource-name>)  [unwired: 7 in]
            n464 = case shown="5" w900 {
              tunnel: w903 -> [w913 w919]
              tunnel: [w909 w915] -> w901
              tunnel: w902 -> [w912 w916]
              tunnel: [w910 w916] -> _
              frame 0, Default {
                w908 = u16 1 items=["BF - Lamp", "SOLA"] ("Light Source")
                n465 = call "Set Lamp intensity.vi"("error in (no error)"=w913, "Lamp Intensity (1.0 V)"=0.0, "VISA Resource Name"=w912) -> ("error out"=w909:errorcluster, "VISA Resource Name Out"=w910:refnum<visa-resource-name>)  [unwired: 7 in]
                n466 = local write "Light Source"(w908) -> ()
              }
              frame 5 {
                w914 = u16 0 items=["BF - Lamp", "SOLA"] ("Light Source")
                n467 = call "lm Color Level.vi"("error in (no error)"=w919, "str_Level"="0", "str_Color"="WHITE") -> ("error out"=w915:errorcluster)  [unwired: 6 in, 2 out]
                n468 = local write "Light Source"(w914) -> ()
              }
            }
          }
          frame "FOCUS" {
            n469 = call "Move Focusing Unit.vi"("VISA Resource Name"=w934, "Device Number (1)"=2, "Direction (1: Down)"=enum16{"Up", "Down", "Abs"}."Abs", "Step (0.0 um)"=w930, "error in (no error)"=w933) -> ("VISA Resource Name Out"=w925:refnum<visa-resource-name>, "error out"=w924:errorcluster)  [unwired: 9 in]
            n470 = call "OlympusQuery.vi"("error in (no error)"=w924, "Device Number\n(1: -Condensor\n     - Objective\n     - Lamp\n     - Shutter\n2: - Z-Motion\n   - Autofocus)"=2 ("Device Number\n(1: -Condensor\n     - Objective\n     - Lamp\n     - Shutter\n2: - Z-Motion\n   - Autofocus)"), "String"="POS?", "VISA Resource Name In"=w925) -> ("error out"=w923:errorcluster, "Result"=w929:string)  [unwired: 5 in, 1 out]
            n471 = Decimal String To Number(string=w929, default (0L)=0.0 ("default (0 I32)")) -> (number=w922:dbl)  [unwired: 1 in, 1 out]
            n472 = Divide(x=w922, y=1000.0) -> (x/y=w921:dbl)
            n473 = local write "Focus [um]"(w921) -> ()
          }
          frame "INTENSITY" {
            n474 = local read "Light Source"() -> (w939:u16)
            n475 = case shown="0, Default" w939 {
              tunnel: w938 -> [w949 w959]
              tunnel: w937 -> [_ w957]
              tunnel: w936 -> [w950 w955]
              tunnel: [w940 w954] -> w935
              frame 1 {
                n476 = Number To Decimal String(number=w949) -> (decimal integer string=w948:string)  [unwired: 1 in]
                n477 = local read "Enable Lamp"() -> (w951:bool)
                n478 = call "lm Color Level.vi"("error in (no error)"=w950, "str_Level"=w948, "str_Color"="WHITE") -> ("error out"=w942:errorcluster, "str_Color out"=w941:string)  [unwired: 6 in, 1 out]
                n479 = Greater Than 0?(x=w949) -> (x > 0?=w952:bool)
                n480 = And(x=w952, y=w951) -> (x .and. y?=w947:bool)
                n481 = Boolean To (0,1)(Boolean=w947) -> (0, 1=w945:i16)
                n482 = Index Array(array=string[] ["OFF", "ON"], index=w945) -> (element=w944:string)
                n483 = call "lm Color Enable.vi"("error in (no error)"=w942, "str_State"=w944, "str_Color"=w941) -> ("error out"=w940:errorcluster)  [unwired: 6 in, 2 out]
              }
              frame 0, Default {
                n484 = local read "Lamp Type (0: Transmitted)"() -> (w953:enum16{"Transmitted", "Reflected"})
                n485 = Multiply(x=w959, y=0.12) -> (x*y=w956:dbl)
                n486 = call "Configure Lamp.vi"("VISA Resource Name"=w957, "Lamp Intensity (1.0 V)"=w956, "Lamp Type (0: Transmitted)"=w953, "error in (no error)"=w955) -> ("error out"=w954:errorcluster)  [unwired: 10 in, 1 out]
              }
            }
          }
          frame "OBJECTIVE" {
            n487 = To Unsigned Long Integer(number=w961) -> (unsigned 32bit integer=w963:u32)
            n488 = Increment(x=w963) -> (x+1=w962:u32)
            n489 = call "Set Active Objective.vi"("error in (no error)"=w964, "Objective Number (1)"=w962, "VISA Resource Name"=w960) -> ("error out"=w965:errorcluster)  [unwired: 7 in, 1 out]
          }
          frame "FOCUSUPDATE" {
            n490 = call "OlympusQuery.vi"("error in (no error)"=w967, "Device Number\n(1: -Condensor\n     - Objective\n     - Lamp\n     - Shutter\n2: - Z-Motion\n   - Autofocus)"=2 ("Device Number\n(1: -Condensor\n     - Objective\n     - Lamp\n     - Shutter\n2: - Z-Motion\n   - Autofocus)"), "String"="POS?", "VISA Resource Name In"=w966) -> ("Result"=w972:string)  [unwired: 5 in, 2 out]
            n491 = Decimal String To Number(string=w972, default (0L)=0.0 ("default (0 I32)")) -> (number=w973:dbl)  [unwired: 1 in, 1 out]
            n492 = Divide(x=w973, y=1000.0) -> (x/y=w974:dbl)
            n493 = local write "Focus [um]"(w974) -> ()
          }
          frame "PRISM" {
            n494 = local read "Prism Position (1: Bi)"() -> (w978:enum16{"Bi", "Side"})
            n495 = To Unsigned Long Integer(number=w978) -> (unsigned 32bit integer=w979:u32)
            n496 = call "Select Prism.vi"("error in (no error)"=w975, "Prism Position (0: Bi)"=w979, "VISA Resource Name"=w976) -> ("error out"=w977:errorcluster)  [unwired: 7 in, 1 out]
          }
          frame "SHUTTER" {
            n497 = call "Set Shutter Status Extended.vi"("VISA Resource Name"=w980, "Shutter Status (0: Open)"=w981, "error in (no error)"=w982) -> ("error out"=w983:errorcluster)  [unwired: 11 in, 1 out]
          }
          frame "", Default {
            n498 = Merge Errors(errorcluster {"status"=FALSE, "code"=9999, "source"="Unknown Element in the queue"} ("error constant"), w984) -> (w985:errorcluster)
          }
          frame "SOLA ENABLE" {
            n499 = Not Equal To 0?(x=w991) -> (x != 0?=w990:bool)
            n500 = local read "Intensity [%]"() -> (w988:dbl)
            n501 = Boolean To (0,1)(Boolean=w990) -> (0, 1=w997:i16)
            n502 = Index Array(array=string[] ["OFF", "ON"], index=w997) -> (element=w989:string)
            n503 = Number To Decimal String(number=w988) -> (decimal integer string=w994:string)  [unwired: 1 in]
            n504 = call "lm Color Enable.vi"("error in (no error)"=w993, "str_State"=w989, "str_Color"="WHITE") -> ("error out"=w996:errorcluster, "str_Color out"=w995:string)  [unwired: 6 in, 1 out]
            n505 = call "lm Color Level.vi"("error in (no error)"=w996, "str_Level"=w994, "str_Color"=w995) -> ("error out"=w987:errorcluster)  [unwired: 6 in, 2 out]
          }
        }
      }
      n506 = while {
        shift-right: [w1000] -> w217
        shift-left: w242 -> [w1002]
        tunnel: w243 -> [w1003]
        tunnel: [w1007] -> w218
        stop <- w1006 stop-if-true
        # "Microscope Control Queue"
        n507 = event shown="[3] \"Intensity [%]\": Value Change" {
          selector: _ -> [_ _ _ _ _ _ _ _ _]
          dyn-events: _ -> [_ _ _ _ _ _ _ _ _]
          timeout: 0 -> [_ _ _ _ _ _ _ _ _]
          tunnel: w1002 -> [w1017 w1026 w1035 w1064 w1074 w1082 w1087 w1096 w1101]
          tunnel: [w1016 w1025 w1033 w1062 w1072 w1080 w1085 w1094 w1099] -> w1001
          tunnel: w1003 -> [w1018 w1027 w1036 w1065 w1075 w1083 w1088 w1097 w1102]
          tunnel: [w1015 w1024 w1032 w1063 w1073 w1081 w1086 w1095 w1100] -> w1007
          event Timeout {
            n508 = event-data() -> ()  [unwired: 1 in, 3 out]
            n509 = Get Queue Status(queue=w1018, return elements? (F)=TRUE, error in (no error)=w1017) -> (queue out=w1015:refnum<queue>, error out=w1016:errorcluster, elements=→"elements":cluster{"Button":string, "Value":dbl}[])  [unwired: 5 out]
          }
          event "Enable Lamp": Value Change {
            n510 = event-data() -> ("NewVal"=w1020:bool)  [unwired: 1 in, 5 out]
            n511 = local read "Light Source"() -> (w1023:u16)
            n512 = case shown="0, Default" w1023 {
              tunnel: ["BF ENABLE" "SOLA ENABLE"] -> w1022
              frame 0, Default {
              }
              frame 1 {
              }
            }
            n513 = case shown="True" w1020 {
              tunnel: [0.0 1.0] -> w1019
              frame False {
              }
              frame True {
              }
            }
            n514 = Bundle(w1022, w1019) -> (w1021:cluster{string, dbl})  [unwired: 1 in]
            n515 = Enqueue Element(queue=w1027, element=w1021, error in (no error)=w1026) -> (queue out=w1024:refnum<queue>, error out=w1025:errorcluster)  [unwired: 1 in, 1 out]
          }
          event "Light Source": Value Change {
            n516 = event-data() -> ("NewVal"=w1034:u16)  [unwired: 1 in, 5 out]
            n517 = case shown="1" w1034 {
              tunnel: w1036 -> [w1048 w1060]
              tunnel: w1035 -> [w1047 w1059]
              tunnel: [w1044 w1056] -> w1033
              tunnel: [w1043 w1055] -> w1032
              frame 0, Default {
                n518 = Bundle("Button"="SOLA ENABLE", "Value"=0.0) -> (w1040:cluster{"Button":string, "Value":dbl})  [unwired: 1 in]
                n519 = Enqueue Element(queue=w1048, element=w1040, error in (no error)=w1047) -> (queue out=w1046:refnum<queue>, error out=w1045:errorcluster)  [unwired: 1 in, 1 out]
                n520 = Bundle("Button"="BF ENABLE", "Value"=1.0) -> (w1037:cluster{"Button":string, "Value":dbl})  [unwired: 1 in]
                n521 = Enqueue Element(queue=w1046, element=w1037, error in (no error)=w1045) -> (queue out=w1043:refnum<queue>, error out=w1044:errorcluster)  [unwired: 1 in, 1 out]
              }
              frame 1 {
                n522 = Bundle("Button"="BF ENABLE", "Value"=0.0) -> (w1052:cluster{"Button":string, "Value":dbl})  [unwired: 1 in]
                n523 = Enqueue Element(queue=w1060, element=w1052, error in (no error)=w1059) -> (queue out=w1058:refnum<queue>, error out=w1057:errorcluster)  [unwired: 1 in, 1 out]
                n524 = Bundle("Button"="SOLA ENABLE", "Value"=1.0) -> (w1049:cluster{"Button":string, "Value":dbl})  [unwired: 1 in]
                n525 = Enqueue Element(queue=w1058, element=w1049, error in (no error)=w1057) -> (queue out=w1055:refnum<queue>, error out=w1056:errorcluster)  [unwired: 1 in, 1 out]
              }
            }
          }
          event "Intensity [%]": Value Change {
            n526 = event-data() -> ("NewVal"=w1066:dbl)  [unwired: 1 in, 5 out]
            n527 = Bundle("INTENSITY", "NewVal"=w1066) -> (w1061:cluster{string, "NewVal":dbl})  [unwired: 1 in]
            n528 = Enqueue Element(queue=w1065, element=w1061, error in (no error)=w1064) -> (queue out=w1063:refnum<queue>, error out=w1062:errorcluster)  [unwired: 1 in, 1 out]
          }
          event "Prism Position (1: Bi)": Value Change {
            n529 = event-data() -> ("NewVal"=w1070:enum16{"Bi", "Side"})  [unwired: 1 in, 5 out]
            n530 = To Double Precision Float(number=w1070) -> (double precision float=w1068:dbl)
            n531 = Bundle("PRISM", w1068) -> (w1069:cluster{string, dbl})  [unwired: 1 in]
            n532 = Enqueue Element(queue=w1075, element=w1069, error in (no error)=w1074) -> (queue out=w1073:refnum<queue>, error out=w1072:errorcluster)  [unwired: 1 in, 1 out]
          }
          event "Shutter": Value Change {
            n533 = event-data() -> ("NewVal"=w1079:bool)  [unwired: 1 in, 5 out]
            n534 = Boolean To (0,1)(Boolean=w1079) -> (0, 1=w1078:i16)
            n535 = Bundle("SHUTTER", w1078) -> (w1076:cluster{string, i16})  [unwired: 1 in]
            n536 = Enqueue Element(queue=w1083, element=w1076, error in (no error)=w1082) -> (queue out=w1081:refnum<queue>, error out=w1080:errorcluster)  [unwired: 1 in, 1 out]
          }
          event "Objective": Value Change {
            n537 = event-data() -> ("NewVal"=w1090:enum16{"x 4", "x 10", "x 20", "x 40", "x 100"})  [unwired: 1 in, 5 out]
            n538 = Bundle("OBJECTIVE", "NewVal"=w1090) -> (w1084:T14)  [unwired: 1 in]
            n539 = Enqueue Element(queue=w1088, element=w1084, error in (no error)=w1087) -> (queue out=w1086:refnum<queue>, error out=w1085:errorcluster)  [unwired: 1 in, 1 out]
          }
          event "Focus [um]": Value Change {
            n540 = event-data() -> ("NewVal"=w1092:dbl)  [unwired: 1 in, 5 out]
            n541 = Bundle("FOCUS", "NewVal"=w1092) -> (w1091:cluster{string, "NewVal":dbl})  [unwired: 1 in]
            n542 = Enqueue Element(queue=w1097, element=w1091, error in (no error)=w1096) -> (queue out=w1095:refnum<queue>, error out=w1094:errorcluster)  [unwired: 1 in, 1 out]
          }
          event "Filter": Value Change {
            n543 = event-data() -> ("NewVal"=w1103:u16)  [unwired: 1 in, 5 out]
            n544 = Bundle("FILTER", "NewVal"=w1103) -> (w1098:cluster{string, "NewVal":u16})  [unwired: 1 in]
            n545 = Enqueue Element(queue=w1102, element=w1098, error in (no error)=w1101) -> (queue out=w1100:refnum<queue>, error out=w1099:errorcluster)  [unwired: 1 in, 1 out]
          }
        }
        n546 = event shown="[0] Timeout" {
          selector: _ -> [_]
          dyn-events: _ -> [_]
          timeout: 100 -> [_]
          tunnel: w1003 -> [w1012]
          tunnel: w1002 -> [w1011]
          tunnel: [w1010] -> w999
          event Timeout {
            n547 = event-data() -> ()  [unwired: 1 in, 3 out]
            n548 = Enqueue Element(queue=w1012, element=cluster{"Button":string, "Value":dbl} {"Button"="FOCUSUPDATE", "Value"=0.0}, error in (no error)=w1011) -> (error out=w1010:errorcluster)  [unwired: 1 in, 2 out]
          }
        }
        n549 = local read "stop"() -> (w1005:bool)
        n550 = Merge Errors(w999, w1001) -> (w1000:errorcluster)
        n551 = Or(x=w1000, y=w1005) -> (x .or. y?=w1006:bool)
      }
      n552 = Flush Queue(queue=w218, error in (no error)=w217) -> (queue out=w220:refnum<queue>, error out=w219:errorcluster)  [unwired: 1 out]
      n553 = Release Queue(queue=w220, force destroy? (F)=TRUE, error in (no error)=w219) -> (error out=w231:errorcluster)  [unwired: 2 out]
      n554 = Merge Errors(w231, w232, w222) -> (w233:errorcluster)
    }
    frame #4 {
      w1125 = u32 20002  # DRV Return Success
      n555 = local read "LINX Resource"() -> (w1113:T1)
      n556 = local read "TANGO ID"() -> (w1105:i32)
      n557 = local read "IX 81 Port"() -> (w1116:refnum<visa-resource-name>)
      n558 = local read "SOLA ID"() -> (w1111:u32)
      n559 = call "Logout Device.vi"("Device Number (1)"=1, "VISA Resource Name"=w1116) -> ("error out"=w1117:errorcluster, "VISA Resource Name Out"=w1121:refnum<visa-resource-name>)  [unwired: 8 in]
      n560 = call <vilib>:"Close.vi"("LINX Resource"=w1113) -> ("Error Out"=w1114:errorcluster)  [unwired: 10 in]
      n561 = call "lm Shut Down.vi"("hSerial"=w1111) -> ("error out"=w1112:errorcluster)  [unwired: 9 in, 1 out]
      n562 = call "Shut Down.vi"() -> ("function return"=w1123:u32)  [unwired: 11 in]
      n563 = call "Disconnect.vi"("lLSID"=w1105) -> ("error out"=w1106:errorcluster)  [unwired: 1 in]
      n564 = call "AndorCreaterErrorCluster.vi"() -> ("Array"=w1107:cluster{i32, string}[])  [unwired: 11 in]
      n565 = call "Logout Device.vi"("error in (no error)"=w1117, "Device Number (1)"=2, "VISA Resource Name"=w1121) -> ("error out"=w1118:errorcluster, "VISA Resource Name Out"=w1122:refnum<visa-resource-name>)  [unwired: 7 in]
      n566 = Not Equal?(x=w1125, y=w1123) -> (x != y?=w1124:bool)
      n567 = call <vilib>:"Close.vi"("VISA Resource Name"=w1122, "error in (no error)"=w1118) -> ("error out"=w1115:errorcluster)  [unwired: 13 in]
      n568 = case shown="True" w1124 {
        tunnel: w1123 -> [_ w1134]
        tunnel: w1107 -> [_ w1133]
        tunnel: [errorcluster {"status"=FALSE, "code"=0, "source"=""} ("error constant") w1128] -> w1110
        frame False {
        }
        frame True {
          n569 = call "ConvertErrCodeToMessage.vi"("function return"=w1134, "Array"=w1133) -> ("Element Return"=w1132:cluster{i32, string})  [unwired: 8 in, 1 out]
          n570 = Unbundle(w1132) -> (w1130:i32, w1131:string)
          n571 = Bundle By Name(cluster=errorcluster {"status"=FALSE, "code"=0, "source"=""} ("error constant"), "status"=TRUE, "code"=w1130, "source"=w1131) -> (w1128:errorcluster)
        }
      }
      n572 = Merge Errors(w1109, w1115, w1114, w1112, w1106, w1110) -> (w1108:errorcluster)
    }
    frame #5 {
      n573 = property on="stop" class="Bool (strict)"("Val(Sgnl)"=FALSE ("Value (Signaling)")) -> ()  [unwired: 2 in, 2 out]
    }
  }
  "error out" <- w3
